vi "Read Tiff File (Bitmiracle libtiff.net)_v2.vi"(8 "error in (no error)":errorcluster, 11 "Input path":path=path "C:/0_DLPGUI_V2/lowResTest.tif") -> (0 "error out":errorcluster, 2 "ImageData":T1)   [LabVIEW 2022 SP3]
doc: "This SubVI is a modified version of the file Read Tiff File.vi that is included in the libtiff2.llb library. The libtiff2.llb was provided by Nico_MPI on the NI LabVIEW discussion forum at http://forums.ni.com/t5/LabVIEW/Labview-libtiff-implementation/td-p/929843/page/2.\n\nRead a multipage TIFF returning an array of images and the total number of frames. This VI closes the file after returning the images array."
uses:
  Classes/TopLevel/Typedefs/TiffImageData--Cluster.ctl
  <vilib>/LVH/i3 JSON/JSON Parsing/Get Object Parameter Files/Get Object Parameter - Object.vi
  <vilib>/LVH/i3 JSON/JSON Parsing/Get Array Value at Index Files/Get Array Value at Index - Array.vi
  C:/Nuget/BitMiracle.LibTiff.NET.2.4.649/lib/net40/BitMiracle.LibTiff.NET.dll
  Nuget/BitMiracle.LibTiff.NET.2.4.649/lib/net40/BitMiracle.LibTiff.NET.dll
  <vilib>/LVH/i3 JSON/i3-json.lvlib
panel:
  out "Numeric":i32
  out "ChannelTargetMaterials":string[](array[string])
  out "MaterialNames":string[](array[string])
  out "error out 2":errorcluster
  out "Subject":string
  out "0 6":T2(plugin-control)
  out "0 5":T2(plugin-control)
  out "0 4":T2(plugin-control)
  out "0 3":T2(plugin-control)
  out "0 2":T2(plugin-control)
  out "ScanLineSize":i32
  out "0":T2(plugin-control)
  out "element 2":i32
  out "element":i32
  # "278x1271"
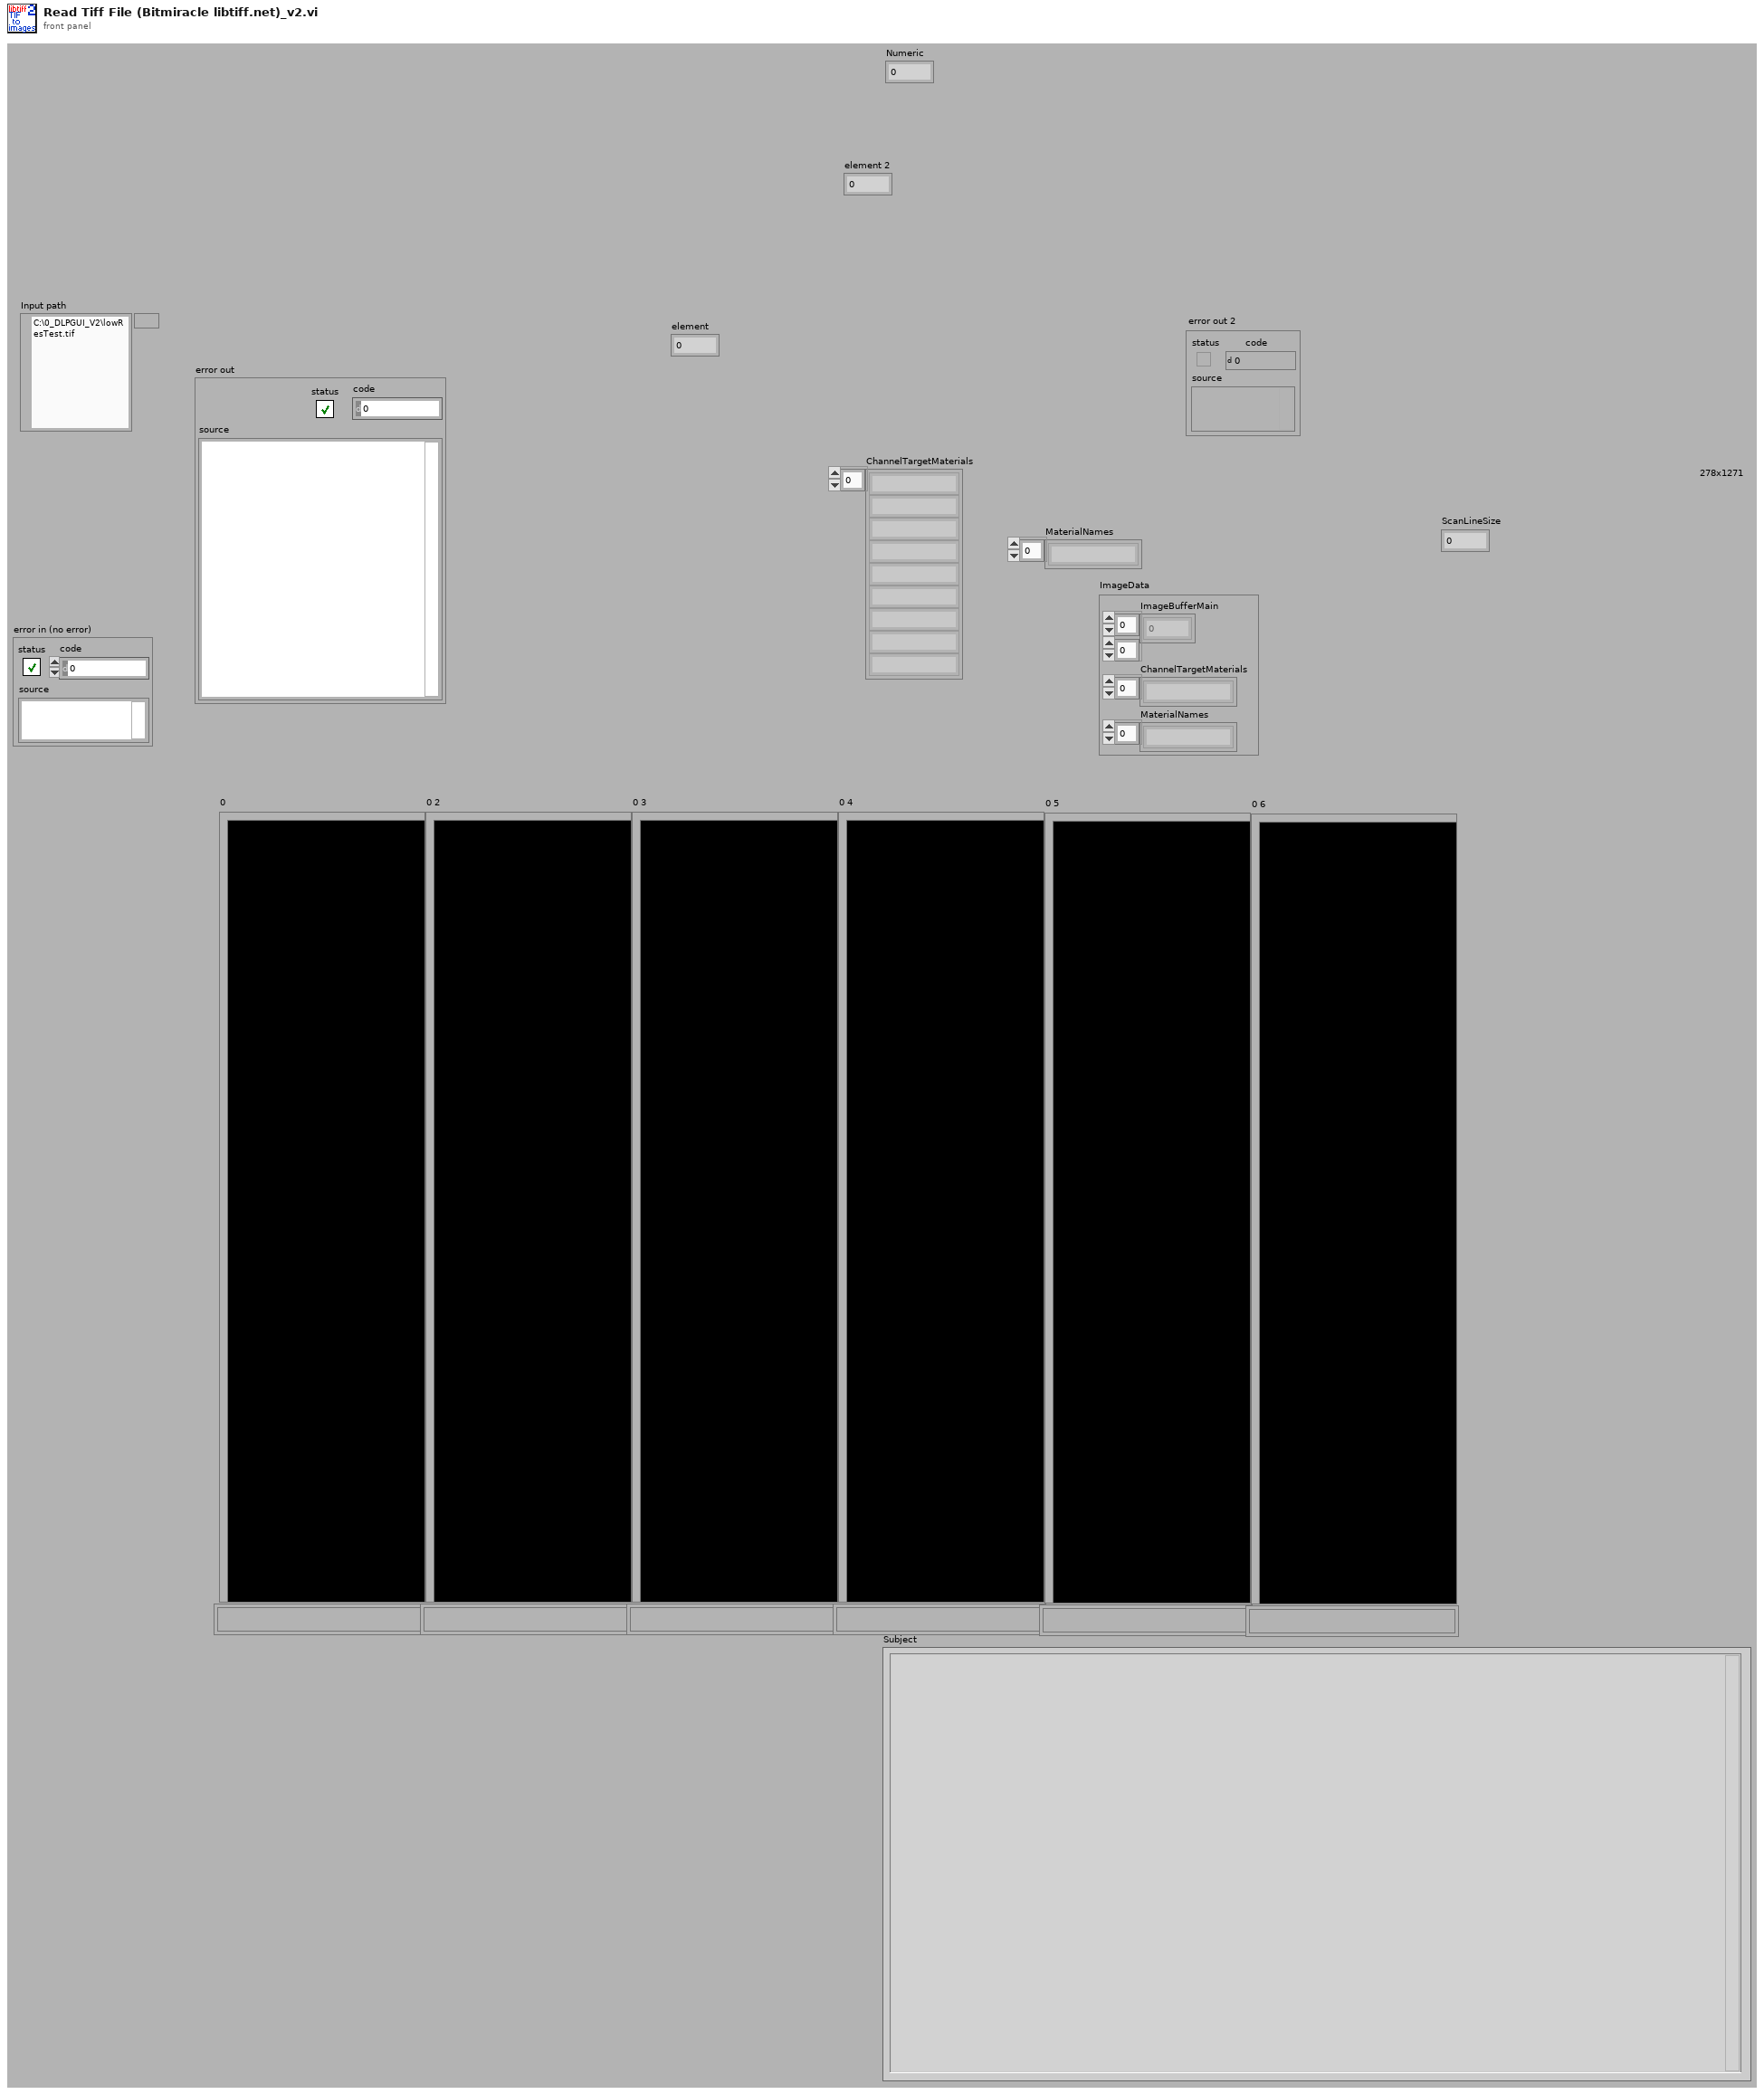
[diagram p1: front panel]
types:
  T1 = typedef "TiffImageData--Cluster.ctl" = cluster{"ImageBufferMain":u8[][], "ChannelTargetMaterials":string[], "MaterialNames":string[]}
  T2 = typedef "IMAQ Image.ctl" = refnum<image>
  T3 = typedef "Image Type" = u32
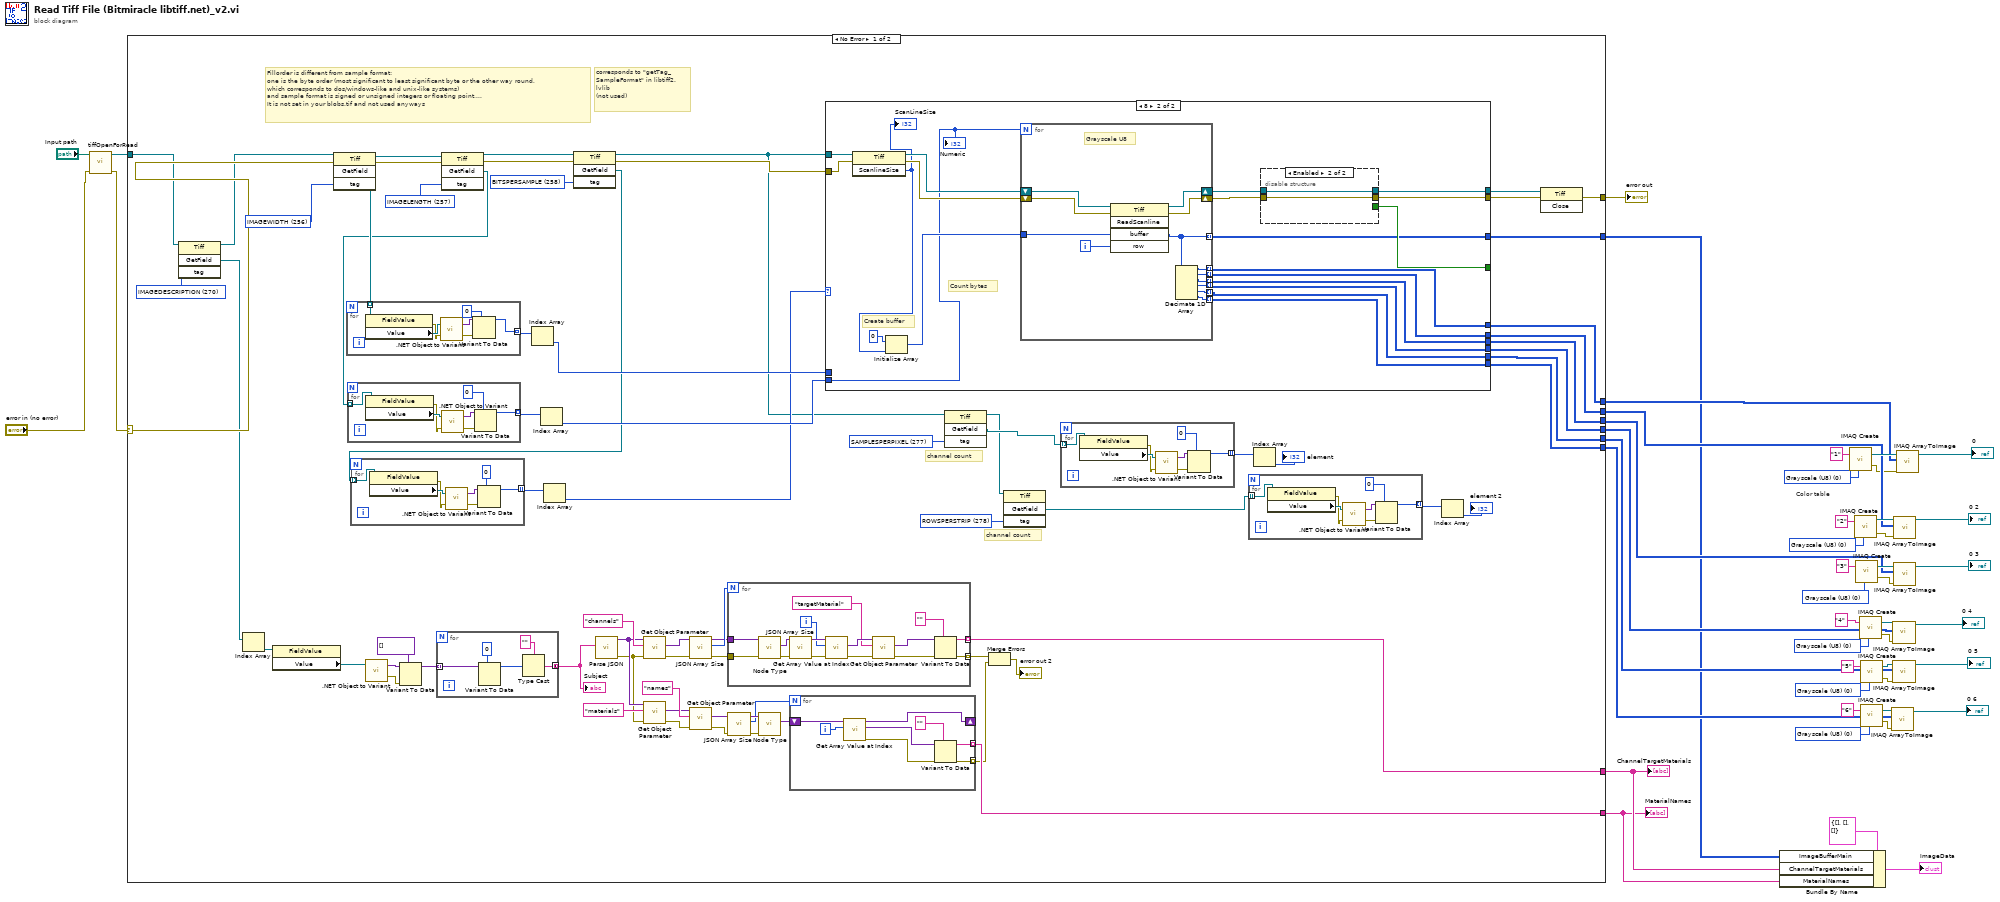
[diagram p0: block diagram]
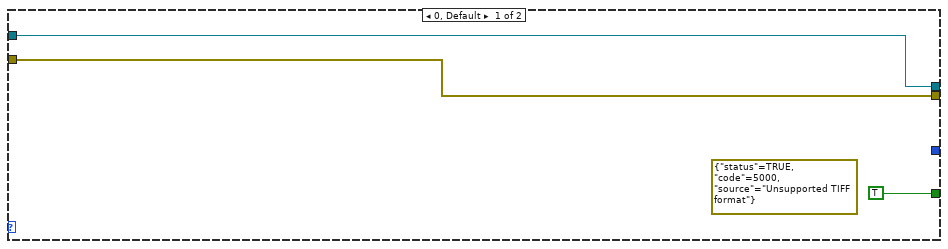
[diagram p2: hidden frame]
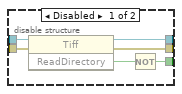
[diagram p3: hidden frame]
diagram:
  w27 = T3 0 items=["Grayscale (U8)", "Grayscale (I16)", "Grayscale (SGL)", "Complex (CSG)", "RGB (U32)", "HSL (U32)", "RGB (U64)", "Grayscale (U16)"] ("Image Type")
  w32 = T3 0 items=["Grayscale (U8)", "Grayscale (I16)", "Grayscale (SGL)", "Complex (CSG)", "RGB (U32)", "HSL (U32)", "RGB (U64)", "Grayscale (U16)"] ("Image Type")
  w29 = T3 0 items=["Grayscale (U8)", "Grayscale (I16)", "Grayscale (SGL)", "Complex (CSG)", "RGB (U32)", "HSL (U32)", "RGB (U64)", "Grayscale (U16)"] ("Image Type")
  w33 = T3 0 items=["Grayscale (U8)", "Grayscale (I16)", "Grayscale (SGL)", "Complex (CSG)", "RGB (U32)", "HSL (U32)", "RGB (U64)", "Grayscale (U16)"] ("Image Type")
  w36 = T3 0 items=["Grayscale (U8)", "Grayscale (I16)", "Grayscale (SGL)", "Complex (CSG)", "RGB (U32)", "HSL (U32)", "RGB (U64)", "Grayscale (U16)"] ("Image Type")
  w40 = T3 0 items=["Grayscale (U8)", "Grayscale (I16)", "Grayscale (SGL)", "Complex (CSG)", "RGB (U32)", "HSL (U32)", "RGB (U64)", "Grayscale (U16)"] ("Image Type")
  # "Color table"
  n1 = call "tiffOpenForRead.vi"("error in (no error)"="error in (no error)", "Path"="Input path") -> ("error out"=w42:errorcluster, "BitMiracle.LibTiff.Classic.Tiff"=w44:refnum<k24>)  [unwired: 8 in]
  n2 = case shown="No Error" w42 {
    selector: w42 -> [w118 w226]
    tunnel: [w114 w226] -> w46
    tunnel: w44 -> [w117 _]
    tunnel: [w113 _] -> w37
    tunnel: [w112 _] -> w24
    tunnel: [w111 _] -> w9
    tunnel: [w110 _] -> w8
    tunnel: [w109 _] -> w7
    tunnel: [w108 _] -> w6
    tunnel: [w107 _] -> w3
    tunnel: [w106 _] -> w2
    tunnel: [w105 _] -> w1
    frame No Error {
      w77 = 270 items=["IGNORE"=0, "SUBFILETYPE"=254, "OSUBFILETYPE"=255, "IMAGEWIDTH"=256, "IMAGELENGTH"=257, "BITSPERSAMPLE"=258, "COMPRESSION"=259, "PHOTOMETRIC"=262, "THRESHHOLDING"=263, "CELLWIDTH"=264, "CELLLENGTH"=265, "FILLORDER"=266, "DOCUMENTNAME"=269, "IMAGEDESCRIPTION"=270, "MAKE"=271, "MODEL"=272, "STRIPOFFSETS"=273, "ORIENTATION"=274, "SAMPLESPERPIXEL"=277, "ROWSPERSTRIP"=278, "STRIPBYTECOUNTS"=279, "MINSAMPLEVALUE"=280, "MAXSAMPLEVALUE"=281, "XRESOLUTION"=282, "YRESOLUTION"=283, "PLANARCONFIG"=284, "PAGENAME"=285, "XPOSITION"=286, "YPOSITION"=287, "FREEOFFSETS"=288, "FREEBYTECOUNTS"=289, "GRAYRESPONSEUNIT"=290, "GRAYRESPONSECURVE"=291, "GROUP3OPTIONS, T4OPTIONS"=292, "GROUP4OPTIONS, T6OPTIONS"=293, "RESOLUTIONUNIT"=296, "PAGENUMBER"=297, "COLORRESPONSEUNIT"=300, "TRANSFERFUNCTION"=301, "SOFTWARE"=305, "DATETIME"=306, "ARTIST"=315, "HOSTCOMPUTER"=316, "PREDICTOR"=317, "WHITEPOINT"=318, "PRIMARYCHROMATICITIES"=319, "COLORMAP"=320, "HALFTONEHINTS"=321, "TILEWIDTH"=322, "TILELENGTH"=323, "TILEOFFSETS"=324, "TILEBYTECOUNTS"=325, "BADFAXLINES"=326, "CLEANFAXDATA"=327, "CONSECUTIVEBADFAXLINES"=328, "SUBIFD"=330, "INKSET"=332, "INKNAMES"=333, "NUMBEROFINKS"=334, "DOTRANGE"=336, "TARGETPRINTER"=337, "EXTRASAMPLES"=338, "SAMPLEFORMAT"=339, "SMINSAMPLEVALUE"=340, "SMAXSAMPLEVALUE"=341, "CLIPPATH"=343, "XCLIPPATHUNITS"=344, "YCLIPPATHUNITS"=345, "INDEXED"=346, "JPEGTABLES"=347, "OPIPROXY"=351, "JPEGPROC"=512, "JPEGIFOFFSET"=513, "JPEGIFBYTECOUNT"=514, "JPEGRESTARTINTERVAL"=515, "JPEGLOSSLESSPREDICTORS"=517, "JPEGPOINTTRANSFORM"=518, "JPEGQTABLES"=519, "JPEGDCTABLES"=520, "JPEGACTABLES"=521, "YCBCRCOEFFICIENTS"=529, "YCBCRSUBSAMPLING"=530, "YCBCRPOSITIONING"=531, "REFERENCEBLACKWHITE"=532, "XMLPACKET"=700, "OPIIMAGEID"=32781, "REFPTS"=32953, "REGIONTACKPOINT"=32954, "REGIONWARPCORNERS"=32955, "REGIONAFFINE"=32956, "MATTEING"=32995, "DATATYPE"=32996, "IMAGEDEPTH"=32997, "TILEDEPTH"=32998, "PIXAR_IMAGEFULLWIDTH"=33300, "PIXAR_IMAGEFULLLENGTH"=33301, "PIXAR_TEXTUREFORMAT"=33302, "PIXAR_WRAPMODES"=33303, "PIXAR_FOVCOT"=33304, "PIXAR_MATRIX_WORLDTOSCREEN"=33305, "PIXAR_MATRIX_WORLDTOCAMERA"=33306, "WRITERSERIALNUMBER"=33405, "COPYRIGHT"=33432, "EXIF_EXPOSURETIME"=33434, "EXIF_FNUMBER"=33437, "GEOTIFF_MODELPIXELSCALETAG"=33550, "RICHTIFFIPTC"=33723, "GEOTIFF_MODELTIEPOINTTAG"=33922, "IT8SITE"=34016, "IT8COLORSEQUENCE"=34017, "IT8HEADER"=34018, "IT8RASTERPADDING"=34019, "IT8BITSPERRUNLENGTH"=34020, "IT8BITSPEREXTENDEDRUNLENGTH"=34021, "IT8COLORTABLE"=34022, "IT8IMAGECOLORINDICATOR"=34023, "IT8BKGCOLORINDICATOR"=34024, "IT8IMAGECOLORVALUE"=34025, "IT8BKGCOLORVALUE"=34026, "IT8PIXELINTENSITYRANGE"=34027, "IT8TRANSPARENCYINDICATOR"=34028, "IT8COLORCHARACTERIZATION"=34029, "IT8HCUSAGE"=34030, "IT8TRAPINDICATOR"=34031, "IT8CMYKEQUIVALENT"=34032, "FRAMECOUNT"=34232, "GEOTIFF_MODELTRANSFORMATIONTAG"=34264, "PHOTOSHOP"=34377, "EXIFIFD"=34665, "ICCPROFILE"=34675, "GEOTIFF_GEOKEYDIRECTORYTAG"=34735, "GEOTIFF_GEODOUBLEPARAMSTAG"=34736, "GEOTIFF_GEOASCIIPARAMSTAG"=34737, "JBIGOPTIONS"=34750, "EXIF_EXPOSUREPROGRAM"=34850, "EXIF_SPECTRALSENSITIVITY"=34852, "GPSIFD"=34853, "EXIF_ISOSPEEDRATINGS"=34855, "EXIF_OECF"=34856, "FAXRECVPARAMS"=34908, "FAXSUBADDRESS"=34909, "FAXRECVTIME"=34910, "FAXDCS"=34911, "FEDEX_EDR"=34929, "EXIF_EXIFVERSION"=36864, "EXIF_DATETIMEORIGINAL"=36867, "EXIF_DATETIMEDIGITIZED"=36868, "EXIF_COMPONENTSCONFIGURATION"=37121, "EXIF_COMPRESSEDBITSPERPIXEL"=37122, "EXIF_SHUTTERSPEEDVALUE"=37377, "EXIF_APERTUREVALUE"=37378, "EXIF_BRIGHTNESSVALUE"=37379, "EXIF_EXPOSUREBIASVALUE"=37380, "EXIF_MAXAPERTUREVALUE"=37381, "EXIF_SUBJECTDISTANCE"=37382, "EXIF_METERINGMODE"=37383, "EXIF_LIGHTSOURCE"=37384, "EXIF_FLASH"=37385, "EXIF_FOCALLENGTH"=37386, "EXIF_SUBJECTAREA"=37396, "STONITS"=37439, "EXIF_MAKERNOTE"=37500, "EXIF_USERCOMMENT"=37510, "EXIF_SUBSECTIME"=37520, "EXIF_SUBSECTIMEORIGINAL"=37521, "EXIF_SUBSECTIMEDIGITIZED"=37522, "EXIF_FLASHPIXVERSION"=40960, "EXIF_COLORSPACE"=40961, "EXIF_PIXELXDIMENSION"=40962, "EXIF_PIXELYDIMENSION"=40963, "EXIF_RELATEDSOUNDFILE"=40964, "INTEROPERABILITYIFD"=40965, "EXIF_FLASHENERGY"=41483, "EXIF_SPATIALFREQUENCYRESPONSE"=41484, "EXIF_FOCALPLANEXRESOLUTION"=41486, "EXIF_FOCALPLANEYRESOLUTION"=41487, "EXIF_FOCALPLANERESOLUTIONUNIT"=41488, "EXIF_SUBJECTLOCATION"=41492, "EXIF_EXPOSUREINDEX"=41493, "EXIF_SENSINGMETHOD"=41495, "EXIF_FILESOURCE"=41728, "EXIF_SCENETYPE"=41729, "EXIF_CFAPATTERN"=41730, "EXIF_CUSTOMRENDERED"=41985, "EXIF_EXPOSUREMODE"=41986, "EXIF_WHITEBALANCE"=41987, "EXIF_DIGITALZOOMRATIO"=41988, "EXIF_FOCALLENGTHIN35MMFILM"=41989, "EXIF_SCENECAPTURETYPE"=41990, "EXIF_GAINCONTROL"=41991, "EXIF_CONTRAST"=41992, "EXIF_SATURATION"=41993, "EXIF_SHARPNESS"=41994, "EXIF_DEVICESETTINGDESCRIPTION"=41995, "EXIF_SUBJECTDISTANCERANGE"=41996, "EXIF_IMAGEUNIQUEID"=42016, "DNGVERSION"=50706, "DNGBACKWARDVERSION"=50707, "UNIQUECAMERAMODEL"=50708, "LOCALIZEDCAMERAMODEL"=50709, "CFAPLANECOLOR"=50710, "CFALAYOUT"=50711, "LINEARIZATIONTABLE"=50712, "BLACKLEVELREPEATDIM"=50713, "BLACKLEVEL"=50714, "BLACKLEVELDELTAH"=50715, "BLACKLEVELDELTAV"=50716, "WHITELEVEL"=50717, "DEFAULTSCALE"=50718, "DEFAULTCROPORIGIN"=50719, "DEFAULTCROPSIZE"=50720, "COLORMATRIX1"=50721, "COLORMATRIX2"=50722, "CAMERACALIBRATION1"=50723, "CAMERACALIBRATION2"=50724, "REDUCTIONMATRIX1"=50725, "REDUCTIONMATRIX2"=50726, "ANALOGBALANCE"=50727, "ASSHOTNEUTRAL"=50728, "ASSHOTWHITEXY"=50729, "BASELINEEXPOSURE"=50730, "BASELINENOISE"=50731, "BASELINESHARPNESS"=50732, "BAYERGREENSPLIT"=50733, "LINEARRESPONSELIMIT"=50734, "CAMERASERIALNUMBER"=50735, "LENSINFO"=50736, "CHROMABLURRADIUS"=50737, "ANTIALIASSTRENGTH"=50738, "SHADOWSCALE"=50739, "DNGPRIVATEDATA"=50740, "MAKERNOTESAFETY"=50741, "CALIBRATIONILLUMINANT1"=50778, "CALIBRATIONILLUMINANT2"=50779, "BESTQUALITYSCALE"=50780, "RAWDATAUNIQUEID"=50781, "ORIGINALRAWFILENAME"=50827, "ORIGINALRAWFILEDATA"=50828, "ACTIVEAREA"=50829, "MASKEDAREAS"=50830, "ASSHOTICCPROFILE"=50831, "ASSHOTPREPROFILEMATRIX"=50832, "CURRENTICCPROFILE"=50833, "CURRENTPREPROFILEMATRIX"=50834, "DCSHUESHIFTVALUES"=65535, "FAXMODE"=65536, "JPEGQUALITY"=65537, "JPEGCOLORMODE"=65538, "JPEGTABLESMODE"=65539, "FAXFILLFUNC"=65540, "PIXARLOGDATAFMT"=65549, "DCSIMAGERTYPE"=65550, "DCSINTERPMODE"=65551, "DCSBALANCEARRAY"=65552, "DCSCORRECTMATRIX"=65553, "DCSGAMMA"=65554, "DCSTOESHOULDERPTS"=65555, "DCSCALIBRATIONFD"=65556, "ZIPQUALITY"=65557, "PIXARLOGQUALITY"=65558, "DCSCLIPRECTANGLE"=65559, "SGILOGDATAFMT"=65560, "SGILOGENCODE"=65561] ("tag")
      w82 = 278 items=["IGNORE"=0, "SUBFILETYPE"=254, "OSUBFILETYPE"=255, "IMAGEWIDTH"=256, "IMAGELENGTH"=257, "BITSPERSAMPLE"=258, "COMPRESSION"=259, "PHOTOMETRIC"=262, "THRESHHOLDING"=263, "CELLWIDTH"=264, "CELLLENGTH"=265, "FILLORDER"=266, "DOCUMENTNAME"=269, "IMAGEDESCRIPTION"=270, "MAKE"=271, "MODEL"=272, "STRIPOFFSETS"=273, "ORIENTATION"=274, "SAMPLESPERPIXEL"=277, "ROWSPERSTRIP"=278, "STRIPBYTECOUNTS"=279, "MINSAMPLEVALUE"=280, "MAXSAMPLEVALUE"=281, "XRESOLUTION"=282, "YRESOLUTION"=283, "PLANARCONFIG"=284, "PAGENAME"=285, "XPOSITION"=286, "YPOSITION"=287, "FREEOFFSETS"=288, "FREEBYTECOUNTS"=289, "GRAYRESPONSEUNIT"=290, "GRAYRESPONSECURVE"=291, "GROUP3OPTIONS, T4OPTIONS"=292, "GROUP4OPTIONS, T6OPTIONS"=293, "RESOLUTIONUNIT"=296, "PAGENUMBER"=297, "COLORRESPONSEUNIT"=300, "TRANSFERFUNCTION"=301, "SOFTWARE"=305, "DATETIME"=306, "ARTIST"=315, "HOSTCOMPUTER"=316, "PREDICTOR"=317, "WHITEPOINT"=318, "PRIMARYCHROMATICITIES"=319, "COLORMAP"=320, "HALFTONEHINTS"=321, "TILEWIDTH"=322, "TILELENGTH"=323, "TILEOFFSETS"=324, "TILEBYTECOUNTS"=325, "BADFAXLINES"=326, "CLEANFAXDATA"=327, "CONSECUTIVEBADFAXLINES"=328, "SUBIFD"=330, "INKSET"=332, "INKNAMES"=333, "NUMBEROFINKS"=334, "DOTRANGE"=336, "TARGETPRINTER"=337, "EXTRASAMPLES"=338, "SAMPLEFORMAT"=339, "SMINSAMPLEVALUE"=340, "SMAXSAMPLEVALUE"=341, "CLIPPATH"=343, "XCLIPPATHUNITS"=344, "YCLIPPATHUNITS"=345, "INDEXED"=346, "JPEGTABLES"=347, "OPIPROXY"=351, "JPEGPROC"=512, "JPEGIFOFFSET"=513, "JPEGIFBYTECOUNT"=514, "JPEGRESTARTINTERVAL"=515, "JPEGLOSSLESSPREDICTORS"=517, "JPEGPOINTTRANSFORM"=518, "JPEGQTABLES"=519, "JPEGDCTABLES"=520, "JPEGACTABLES"=521, "YCBCRCOEFFICIENTS"=529, "YCBCRSUBSAMPLING"=530, "YCBCRPOSITIONING"=531, "REFERENCEBLACKWHITE"=532, "XMLPACKET"=700, "OPIIMAGEID"=32781, "REFPTS"=32953, "REGIONTACKPOINT"=32954, "REGIONWARPCORNERS"=32955, "REGIONAFFINE"=32956, "MATTEING"=32995, "DATATYPE"=32996, "IMAGEDEPTH"=32997, "TILEDEPTH"=32998, "PIXAR_IMAGEFULLWIDTH"=33300, "PIXAR_IMAGEFULLLENGTH"=33301, "PIXAR_TEXTUREFORMAT"=33302, "PIXAR_WRAPMODES"=33303, "PIXAR_FOVCOT"=33304, "PIXAR_MATRIX_WORLDTOSCREEN"=33305, "PIXAR_MATRIX_WORLDTOCAMERA"=33306, "WRITERSERIALNUMBER"=33405, "COPYRIGHT"=33432, "EXIF_EXPOSURETIME"=33434, "EXIF_FNUMBER"=33437, "RICHTIFFIPTC"=33723, "IT8SITE"=34016, "IT8COLORSEQUENCE"=34017, "IT8HEADER"=34018, "IT8RASTERPADDING"=34019, "IT8BITSPERRUNLENGTH"=34020, "IT8BITSPEREXTENDEDRUNLENGTH"=34021, "IT8COLORTABLE"=34022, "IT8IMAGECOLORINDICATOR"=34023, "IT8BKGCOLORINDICATOR"=34024, "IT8IMAGECOLORVALUE"=34025, "IT8BKGCOLORVALUE"=34026, "IT8PIXELINTENSITYRANGE"=34027, "IT8TRANSPARENCYINDICATOR"=34028, "IT8COLORCHARACTERIZATION"=34029, "IT8HCUSAGE"=34030, "IT8TRAPINDICATOR"=34031, "IT8CMYKEQUIVALENT"=34032, "FRAMECOUNT"=34232, "PHOTOSHOP"=34377, "EXIFIFD"=34665, "ICCPROFILE"=34675, "JBIGOPTIONS"=34750, "EXIF_EXPOSUREPROGRAM"=34850, "EXIF_SPECTRALSENSITIVITY"=34852, "GPSIFD"=34853, "EXIF_ISOSPEEDRATINGS"=34855, "EXIF_OECF"=34856, "FAXRECVPARAMS"=34908, "FAXSUBADDRESS"=34909, "FAXRECVTIME"=34910, "FAXDCS"=34911, "FEDEX_EDR"=34929, "EXIF_EXIFVERSION"=36864, "EXIF_DATETIMEORIGINAL"=36867, "EXIF_DATETIMEDIGITIZED"=36868, "EXIF_COMPONENTSCONFIGURATION"=37121, "EXIF_COMPRESSEDBITSPERPIXEL"=37122, "EXIF_SHUTTERSPEEDVALUE"=37377, "EXIF_APERTUREVALUE"=37378, "EXIF_BRIGHTNESSVALUE"=37379, "EXIF_EXPOSUREBIASVALUE"=37380, "EXIF_MAXAPERTUREVALUE"=37381, "EXIF_SUBJECTDISTANCE"=37382, "EXIF_METERINGMODE"=37383, "EXIF_LIGHTSOURCE"=37384, "EXIF_FLASH"=37385, "EXIF_FOCALLENGTH"=37386, "EXIF_SUBJECTAREA"=37396, "STONITS"=37439, "EXIF_MAKERNOTE"=37500, "EXIF_USERCOMMENT"=37510, "EXIF_SUBSECTIME"=37520, "EXIF_SUBSECTIMEORIGINAL"=37521, "EXIF_SUBSECTIMEDIGITIZED"=37522, "EXIF_FLASHPIXVERSION"=40960, "EXIF_COLORSPACE"=40961, "EXIF_PIXELXDIMENSION"=40962, "EXIF_PIXELYDIMENSION"=40963, "EXIF_RELATEDSOUNDFILE"=40964, "INTEROPERABILITYIFD"=40965, "EXIF_FLASHENERGY"=41483, "EXIF_SPATIALFREQUENCYRESPONSE"=41484, "EXIF_FOCALPLANEXRESOLUTION"=41486, "EXIF_FOCALPLANEYRESOLUTION"=41487, "EXIF_FOCALPLANERESOLUTIONUNIT"=41488, "EXIF_SUBJECTLOCATION"=41492, "EXIF_EXPOSUREINDEX"=41493, "EXIF_SENSINGMETHOD"=41495, "EXIF_FILESOURCE"=41728, "EXIF_SCENETYPE"=41729, "EXIF_CFAPATTERN"=41730, "EXIF_CUSTOMRENDERED"=41985, "EXIF_EXPOSUREMODE"=41986, "EXIF_WHITEBALANCE"=41987, "EXIF_DIGITALZOOMRATIO"=41988, "EXIF_FOCALLENGTHIN35MMFILM"=41989, "EXIF_SCENECAPTURETYPE"=41990, "EXIF_GAINCONTROL"=41991, "EXIF_CONTRAST"=41992, "EXIF_SATURATION"=41993, "EXIF_SHARPNESS"=41994, "EXIF_DEVICESETTINGDESCRIPTION"=41995, "EXIF_SUBJECTDISTANCERANGE"=41996, "EXIF_IMAGEUNIQUEID"=42016, "DNGVERSION"=50706, "DNGBACKWARDVERSION"=50707, "UNIQUECAMERAMODEL"=50708, "LOCALIZEDCAMERAMODEL"=50709, "CFAPLANECOLOR"=50710, "CFALAYOUT"=50711, "LINEARIZATIONTABLE"=50712, "BLACKLEVELREPEATDIM"=50713, "BLACKLEVEL"=50714, "BLACKLEVELDELTAH"=50715, "BLACKLEVELDELTAV"=50716, "WHITELEVEL"=50717, "DEFAULTSCALE"=50718, "DEFAULTCROPORIGIN"=50719, "DEFAULTCROPSIZE"=50720, "COLORMATRIX1"=50721, "COLORMATRIX2"=50722, "CAMERACALIBRATION1"=50723, "CAMERACALIBRATION2"=50724, "REDUCTIONMATRIX1"=50725, "REDUCTIONMATRIX2"=50726, "ANALOGBALANCE"=50727, "ASSHOTNEUTRAL"=50728, "ASSHOTWHITEXY"=50729, "BASELINEEXPOSURE"=50730, "BASELINENOISE"=50731, "BASELINESHARPNESS"=50732, "BAYERGREENSPLIT"=50733, "LINEARRESPONSELIMIT"=50734, "CAMERASERIALNUMBER"=50735, "LENSINFO"=50736, "CHROMABLURRADIUS"=50737, "ANTIALIASSTRENGTH"=50738, "SHADOWSCALE"=50739, "DNGPRIVATEDATA"=50740, "MAKERNOTESAFETY"=50741, "CALIBRATIONILLUMINANT1"=50778, "CALIBRATIONILLUMINANT2"=50779, "BESTQUALITYSCALE"=50780, "RAWDATAUNIQUEID"=50781, "ORIGINALRAWFILENAME"=50827, "ORIGINALRAWFILEDATA"=50828, "ACTIVEAREA"=50829, "MASKEDAREAS"=50830, "ASSHOTICCPROFILE"=50831, "ASSHOTPREPROFILEMATRIX"=50832, "CURRENTICCPROFILE"=50833, "CURRENTPREPROFILEMATRIX"=50834, "DCSHUESHIFTVALUES"=65535, "FAXMODE"=65536, "JPEGQUALITY"=65537, "JPEGCOLORMODE"=65538, "JPEGTABLESMODE"=65539, "FAXFILLFUNC"=65540, "PIXARLOGDATAFMT"=65549, "DCSIMAGERTYPE"=65550, "DCSINTERPMODE"=65551, "DCSBALANCEARRAY"=65552, "DCSCORRECTMATRIX"=65553, "DCSGAMMA"=65554, "DCSTOESHOULDERPTS"=65555, "DCSCALIBRATIONFD"=65556, "ZIPQUALITY"=65557, "PIXARLOGQUALITY"=65558, "DCSCLIPRECTANGLE"=65559, "SGILOGDATAFMT"=65560, "SGILOGENCODE"=65561] ("tag")
      w87 = 277 items=["IGNORE"=0, "SUBFILETYPE"=254, "OSUBFILETYPE"=255, "IMAGEWIDTH"=256, "IMAGELENGTH"=257, "BITSPERSAMPLE"=258, "COMPRESSION"=259, "PHOTOMETRIC"=262, "THRESHHOLDING"=263, "CELLWIDTH"=264, "CELLLENGTH"=265, "FILLORDER"=266, "DOCUMENTNAME"=269, "IMAGEDESCRIPTION"=270, "MAKE"=271, "MODEL"=272, "STRIPOFFSETS"=273, "ORIENTATION"=274, "SAMPLESPERPIXEL"=277, "ROWSPERSTRIP"=278, "STRIPBYTECOUNTS"=279, "MINSAMPLEVALUE"=280, "MAXSAMPLEVALUE"=281, "XRESOLUTION"=282, "YRESOLUTION"=283, "PLANARCONFIG"=284, "PAGENAME"=285, "XPOSITION"=286, "YPOSITION"=287, "FREEOFFSETS"=288, "FREEBYTECOUNTS"=289, "GRAYRESPONSEUNIT"=290, "GRAYRESPONSECURVE"=291, "GROUP3OPTIONS, T4OPTIONS"=292, "GROUP4OPTIONS, T6OPTIONS"=293, "RESOLUTIONUNIT"=296, "PAGENUMBER"=297, "COLORRESPONSEUNIT"=300, "TRANSFERFUNCTION"=301, "SOFTWARE"=305, "DATETIME"=306, "ARTIST"=315, "HOSTCOMPUTER"=316, "PREDICTOR"=317, "WHITEPOINT"=318, "PRIMARYCHROMATICITIES"=319, "COLORMAP"=320, "HALFTONEHINTS"=321, "TILEWIDTH"=322, "TILELENGTH"=323, "TILEOFFSETS"=324, "TILEBYTECOUNTS"=325, "BADFAXLINES"=326, "CLEANFAXDATA"=327, "CONSECUTIVEBADFAXLINES"=328, "SUBIFD"=330, "INKSET"=332, "INKNAMES"=333, "NUMBEROFINKS"=334, "DOTRANGE"=336, "TARGETPRINTER"=337, "EXTRASAMPLES"=338, "SAMPLEFORMAT"=339, "SMINSAMPLEVALUE"=340, "SMAXSAMPLEVALUE"=341, "CLIPPATH"=343, "XCLIPPATHUNITS"=344, "YCLIPPATHUNITS"=345, "INDEXED"=346, "JPEGTABLES"=347, "OPIPROXY"=351, "JPEGPROC"=512, "JPEGIFOFFSET"=513, "JPEGIFBYTECOUNT"=514, "JPEGRESTARTINTERVAL"=515, "JPEGLOSSLESSPREDICTORS"=517, "JPEGPOINTTRANSFORM"=518, "JPEGQTABLES"=519, "JPEGDCTABLES"=520, "JPEGACTABLES"=521, "YCBCRCOEFFICIENTS"=529, "YCBCRSUBSAMPLING"=530, "YCBCRPOSITIONING"=531, "REFERENCEBLACKWHITE"=532, "XMLPACKET"=700, "OPIIMAGEID"=32781, "REFPTS"=32953, "REGIONTACKPOINT"=32954, "REGIONWARPCORNERS"=32955, "REGIONAFFINE"=32956, "MATTEING"=32995, "DATATYPE"=32996, "IMAGEDEPTH"=32997, "TILEDEPTH"=32998, "PIXAR_IMAGEFULLWIDTH"=33300, "PIXAR_IMAGEFULLLENGTH"=33301, "PIXAR_TEXTUREFORMAT"=33302, "PIXAR_WRAPMODES"=33303, "PIXAR_FOVCOT"=33304, "PIXAR_MATRIX_WORLDTOSCREEN"=33305, "PIXAR_MATRIX_WORLDTOCAMERA"=33306, "WRITERSERIALNUMBER"=33405, "COPYRIGHT"=33432, "EXIF_EXPOSURETIME"=33434, "EXIF_FNUMBER"=33437, "RICHTIFFIPTC"=33723, "IT8SITE"=34016, "IT8COLORSEQUENCE"=34017, "IT8HEADER"=34018, "IT8RASTERPADDING"=34019, "IT8BITSPERRUNLENGTH"=34020, "IT8BITSPEREXTENDEDRUNLENGTH"=34021, "IT8COLORTABLE"=34022, "IT8IMAGECOLORINDICATOR"=34023, "IT8BKGCOLORINDICATOR"=34024, "IT8IMAGECOLORVALUE"=34025, "IT8BKGCOLORVALUE"=34026, "IT8PIXELINTENSITYRANGE"=34027, "IT8TRANSPARENCYINDICATOR"=34028, "IT8COLORCHARACTERIZATION"=34029, "IT8HCUSAGE"=34030, "IT8TRAPINDICATOR"=34031, "IT8CMYKEQUIVALENT"=34032, "FRAMECOUNT"=34232, "PHOTOSHOP"=34377, "EXIFIFD"=34665, "ICCPROFILE"=34675, "JBIGOPTIONS"=34750, "EXIF_EXPOSUREPROGRAM"=34850, "EXIF_SPECTRALSENSITIVITY"=34852, "GPSIFD"=34853, "EXIF_ISOSPEEDRATINGS"=34855, "EXIF_OECF"=34856, "FAXRECVPARAMS"=34908, "FAXSUBADDRESS"=34909, "FAXRECVTIME"=34910, "FAXDCS"=34911, "FEDEX_EDR"=34929, "EXIF_EXIFVERSION"=36864, "EXIF_DATETIMEORIGINAL"=36867, "EXIF_DATETIMEDIGITIZED"=36868, "EXIF_COMPONENTSCONFIGURATION"=37121, "EXIF_COMPRESSEDBITSPERPIXEL"=37122, "EXIF_SHUTTERSPEEDVALUE"=37377, "EXIF_APERTUREVALUE"=37378, "EXIF_BRIGHTNESSVALUE"=37379, "EXIF_EXPOSUREBIASVALUE"=37380, "EXIF_MAXAPERTUREVALUE"=37381, "EXIF_SUBJECTDISTANCE"=37382, "EXIF_METERINGMODE"=37383, "EXIF_LIGHTSOURCE"=37384, "EXIF_FLASH"=37385, "EXIF_FOCALLENGTH"=37386, "EXIF_SUBJECTAREA"=37396, "STONITS"=37439, "EXIF_MAKERNOTE"=37500, "EXIF_USERCOMMENT"=37510, "EXIF_SUBSECTIME"=37520, "EXIF_SUBSECTIMEORIGINAL"=37521, "EXIF_SUBSECTIMEDIGITIZED"=37522, "EXIF_FLASHPIXVERSION"=40960, "EXIF_COLORSPACE"=40961, "EXIF_PIXELXDIMENSION"=40962, "EXIF_PIXELYDIMENSION"=40963, "EXIF_RELATEDSOUNDFILE"=40964, "INTEROPERABILITYIFD"=40965, "EXIF_FLASHENERGY"=41483, "EXIF_SPATIALFREQUENCYRESPONSE"=41484, "EXIF_FOCALPLANEXRESOLUTION"=41486, "EXIF_FOCALPLANEYRESOLUTION"=41487, "EXIF_FOCALPLANERESOLUTIONUNIT"=41488, "EXIF_SUBJECTLOCATION"=41492, "EXIF_EXPOSUREINDEX"=41493, "EXIF_SENSINGMETHOD"=41495, "EXIF_FILESOURCE"=41728, "EXIF_SCENETYPE"=41729, "EXIF_CFAPATTERN"=41730, "EXIF_CUSTOMRENDERED"=41985, "EXIF_EXPOSUREMODE"=41986, "EXIF_WHITEBALANCE"=41987, "EXIF_DIGITALZOOMRATIO"=41988, "EXIF_FOCALLENGTHIN35MMFILM"=41989, "EXIF_SCENECAPTURETYPE"=41990, "EXIF_GAINCONTROL"=41991, "EXIF_CONTRAST"=41992, "EXIF_SATURATION"=41993, "EXIF_SHARPNESS"=41994, "EXIF_DEVICESETTINGDESCRIPTION"=41995, "EXIF_SUBJECTDISTANCERANGE"=41996, "EXIF_IMAGEUNIQUEID"=42016, "DNGVERSION"=50706, "DNGBACKWARDVERSION"=50707, "UNIQUECAMERAMODEL"=50708, "LOCALIZEDCAMERAMODEL"=50709, "CFAPLANECOLOR"=50710, "CFALAYOUT"=50711, "LINEARIZATIONTABLE"=50712, "BLACKLEVELREPEATDIM"=50713, "BLACKLEVEL"=50714, "BLACKLEVELDELTAH"=50715, "BLACKLEVELDELTAV"=50716, "WHITELEVEL"=50717, "DEFAULTSCALE"=50718, "DEFAULTCROPORIGIN"=50719, "DEFAULTCROPSIZE"=50720, "COLORMATRIX1"=50721, "COLORMATRIX2"=50722, "CAMERACALIBRATION1"=50723, "CAMERACALIBRATION2"=50724, "REDUCTIONMATRIX1"=50725, "REDUCTIONMATRIX2"=50726, "ANALOGBALANCE"=50727, "ASSHOTNEUTRAL"=50728, "ASSHOTWHITEXY"=50729, "BASELINEEXPOSURE"=50730, "BASELINENOISE"=50731, "BASELINESHARPNESS"=50732, "BAYERGREENSPLIT"=50733, "LINEARRESPONSELIMIT"=50734, "CAMERASERIALNUMBER"=50735, "LENSINFO"=50736, "CHROMABLURRADIUS"=50737, "ANTIALIASSTRENGTH"=50738, "SHADOWSCALE"=50739, "DNGPRIVATEDATA"=50740, "MAKERNOTESAFETY"=50741, "CALIBRATIONILLUMINANT1"=50778, "CALIBRATIONILLUMINANT2"=50779, "BESTQUALITYSCALE"=50780, "RAWDATAUNIQUEID"=50781, "ORIGINALRAWFILENAME"=50827, "ORIGINALRAWFILEDATA"=50828, "ACTIVEAREA"=50829, "MASKEDAREAS"=50830, "ASSHOTICCPROFILE"=50831, "ASSHOTPREPROFILEMATRIX"=50832, "CURRENTICCPROFILE"=50833, "CURRENTPREPROFILEMATRIX"=50834, "DCSHUESHIFTVALUES"=65535, "FAXMODE"=65536, "JPEGQUALITY"=65537, "JPEGCOLORMODE"=65538, "JPEGTABLESMODE"=65539, "FAXFILLFUNC"=65540, "PIXARLOGDATAFMT"=65549, "DCSIMAGERTYPE"=65550, "DCSINTERPMODE"=65551, "DCSBALANCEARRAY"=65552, "DCSCORRECTMATRIX"=65553, "DCSGAMMA"=65554, "DCSTOESHOULDERPTS"=65555, "DCSCALIBRATIONFD"=65556, "ZIPQUALITY"=65557, "PIXARLOGQUALITY"=65558, "DCSCLIPRECTANGLE"=65559, "SGILOGDATAFMT"=65560, "SGILOGENCODE"=65561] ("tag")
      w98 = 258 items=["IGNORE"=0, "SUBFILETYPE"=254, "OSUBFILETYPE"=255, "IMAGEWIDTH"=256, "IMAGELENGTH"=257, "BITSPERSAMPLE"=258, "COMPRESSION"=259, "PHOTOMETRIC"=262, "THRESHHOLDING"=263, "CELLWIDTH"=264, "CELLLENGTH"=265, "FILLORDER"=266, "DOCUMENTNAME"=269, "IMAGEDESCRIPTION"=270, "MAKE"=271, "MODEL"=272, "STRIPOFFSETS"=273, "ORIENTATION"=274, "SAMPLESPERPIXEL"=277, "ROWSPERSTRIP"=278, "STRIPBYTECOUNTS"=279, "MINSAMPLEVALUE"=280, "MAXSAMPLEVALUE"=281, "XRESOLUTION"=282, "YRESOLUTION"=283, "PLANARCONFIG"=284, "PAGENAME"=285, "XPOSITION"=286, "YPOSITION"=287, "FREEOFFSETS"=288, "FREEBYTECOUNTS"=289, "GRAYRESPONSEUNIT"=290, "GRAYRESPONSECURVE"=291, "GROUP3OPTIONS, T4OPTIONS"=292, "GROUP4OPTIONS, T6OPTIONS"=293, "RESOLUTIONUNIT"=296, "PAGENUMBER"=297, "COLORRESPONSEUNIT"=300, "TRANSFERFUNCTION"=301, "SOFTWARE"=305, "DATETIME"=306, "ARTIST"=315, "HOSTCOMPUTER"=316, "PREDICTOR"=317, "WHITEPOINT"=318, "PRIMARYCHROMATICITIES"=319, "COLORMAP"=320, "HALFTONEHINTS"=321, "TILEWIDTH"=322, "TILELENGTH"=323, "TILEOFFSETS"=324, "TILEBYTECOUNTS"=325, "BADFAXLINES"=326, "CLEANFAXDATA"=327, "CONSECUTIVEBADFAXLINES"=328, "SUBIFD"=330, "INKSET"=332, "INKNAMES"=333, "NUMBEROFINKS"=334, "DOTRANGE"=336, "TARGETPRINTER"=337, "EXTRASAMPLES"=338, "SAMPLEFORMAT"=339, "SMINSAMPLEVALUE"=340, "SMAXSAMPLEVALUE"=341, "CLIPPATH"=343, "XCLIPPATHUNITS"=344, "YCLIPPATHUNITS"=345, "INDEXED"=346, "JPEGTABLES"=347, "OPIPROXY"=351, "JPEGPROC"=512, "JPEGIFOFFSET"=513, "JPEGIFBYTECOUNT"=514, "JPEGRESTARTINTERVAL"=515, "JPEGLOSSLESSPREDICTORS"=517, "JPEGPOINTTRANSFORM"=518, "JPEGQTABLES"=519, "JPEGDCTABLES"=520, "JPEGACTABLES"=521, "YCBCRCOEFFICIENTS"=529, "YCBCRSUBSAMPLING"=530, "YCBCRPOSITIONING"=531, "REFERENCEBLACKWHITE"=532, "XMLPACKET"=700, "OPIIMAGEID"=32781, "REFPTS"=32953, "REGIONTACKPOINT"=32954, "REGIONWARPCORNERS"=32955, "REGIONAFFINE"=32956, "MATTEING"=32995, "DATATYPE"=32996, "IMAGEDEPTH"=32997, "TILEDEPTH"=32998, "PIXAR_IMAGEFULLWIDTH"=33300, "PIXAR_IMAGEFULLLENGTH"=33301, "PIXAR_TEXTUREFORMAT"=33302, "PIXAR_WRAPMODES"=33303, "PIXAR_FOVCOT"=33304, "PIXAR_MATRIX_WORLDTOSCREEN"=33305, "PIXAR_MATRIX_WORLDTOCAMERA"=33306, "WRITERSERIALNUMBER"=33405, "COPYRIGHT"=33432, "EXIF_EXPOSURETIME"=33434, "EXIF_FNUMBER"=33437, "RICHTIFFIPTC"=33723, "IT8SITE"=34016, "IT8COLORSEQUENCE"=34017, "IT8HEADER"=34018, "IT8RASTERPADDING"=34019, "IT8BITSPERRUNLENGTH"=34020, "IT8BITSPEREXTENDEDRUNLENGTH"=34021, "IT8COLORTABLE"=34022, "IT8IMAGECOLORINDICATOR"=34023, "IT8BKGCOLORINDICATOR"=34024, "IT8IMAGECOLORVALUE"=34025, "IT8BKGCOLORVALUE"=34026, "IT8PIXELINTENSITYRANGE"=34027, "IT8TRANSPARENCYINDICATOR"=34028, "IT8COLORCHARACTERIZATION"=34029, "IT8HCUSAGE"=34030, "IT8TRAPINDICATOR"=34031, "IT8CMYKEQUIVALENT"=34032, "FRAMECOUNT"=34232, "PHOTOSHOP"=34377, "EXIFIFD"=34665, "ICCPROFILE"=34675, "JBIGOPTIONS"=34750, "EXIF_EXPOSUREPROGRAM"=34850, "EXIF_SPECTRALSENSITIVITY"=34852, "GPSIFD"=34853, "EXIF_ISOSPEEDRATINGS"=34855, "EXIF_OECF"=34856, "FAXRECVPARAMS"=34908, "FAXSUBADDRESS"=34909, "FAXRECVTIME"=34910, "FAXDCS"=34911, "FEDEX_EDR"=34929, "EXIF_EXIFVERSION"=36864, "EXIF_DATETIMEORIGINAL"=36867, "EXIF_DATETIMEDIGITIZED"=36868, "EXIF_COMPONENTSCONFIGURATION"=37121, "EXIF_COMPRESSEDBITSPERPIXEL"=37122, "EXIF_SHUTTERSPEEDVALUE"=37377, "EXIF_APERTUREVALUE"=37378, "EXIF_BRIGHTNESSVALUE"=37379, "EXIF_EXPOSUREBIASVALUE"=37380, "EXIF_MAXAPERTUREVALUE"=37381, "EXIF_SUBJECTDISTANCE"=37382, "EXIF_METERINGMODE"=37383, "EXIF_LIGHTSOURCE"=37384, "EXIF_FLASH"=37385, "EXIF_FOCALLENGTH"=37386, "EXIF_SUBJECTAREA"=37396, "STONITS"=37439, "EXIF_MAKERNOTE"=37500, "EXIF_USERCOMMENT"=37510, "EXIF_SUBSECTIME"=37520, "EXIF_SUBSECTIMEORIGINAL"=37521, "EXIF_SUBSECTIMEDIGITIZED"=37522, "EXIF_FLASHPIXVERSION"=40960, "EXIF_COLORSPACE"=40961, "EXIF_PIXELXDIMENSION"=40962, "EXIF_PIXELYDIMENSION"=40963, "EXIF_RELATEDSOUNDFILE"=40964, "INTEROPERABILITYIFD"=40965, "EXIF_FLASHENERGY"=41483, "EXIF_SPATIALFREQUENCYRESPONSE"=41484, "EXIF_FOCALPLANEXRESOLUTION"=41486, "EXIF_FOCALPLANEYRESOLUTION"=41487, "EXIF_FOCALPLANERESOLUTIONUNIT"=41488, "EXIF_SUBJECTLOCATION"=41492, "EXIF_EXPOSUREINDEX"=41493, "EXIF_SENSINGMETHOD"=41495, "EXIF_FILESOURCE"=41728, "EXIF_SCENETYPE"=41729, "EXIF_CFAPATTERN"=41730, "EXIF_CUSTOMRENDERED"=41985, "EXIF_EXPOSUREMODE"=41986, "EXIF_WHITEBALANCE"=41987, "EXIF_DIGITALZOOMRATIO"=41988, "EXIF_FOCALLENGTHIN35MMFILM"=41989, "EXIF_SCENECAPTURETYPE"=41990, "EXIF_GAINCONTROL"=41991, "EXIF_CONTRAST"=41992, "EXIF_SATURATION"=41993, "EXIF_SHARPNESS"=41994, "EXIF_DEVICESETTINGDESCRIPTION"=41995, "EXIF_SUBJECTDISTANCERANGE"=41996, "EXIF_IMAGEUNIQUEID"=42016, "DNGVERSION"=50706, "DNGBACKWARDVERSION"=50707, "UNIQUECAMERAMODEL"=50708, "LOCALIZEDCAMERAMODEL"=50709, "CFAPLANECOLOR"=50710, "CFALAYOUT"=50711, "LINEARIZATIONTABLE"=50712, "BLACKLEVELREPEATDIM"=50713, "BLACKLEVEL"=50714, "BLACKLEVELDELTAH"=50715, "BLACKLEVELDELTAV"=50716, "WHITELEVEL"=50717, "DEFAULTSCALE"=50718, "DEFAULTCROPORIGIN"=50719, "DEFAULTCROPSIZE"=50720, "COLORMATRIX1"=50721, "COLORMATRIX2"=50722, "CAMERACALIBRATION1"=50723, "CAMERACALIBRATION2"=50724, "REDUCTIONMATRIX1"=50725, "REDUCTIONMATRIX2"=50726, "ANALOGBALANCE"=50727, "ASSHOTNEUTRAL"=50728, "ASSHOTWHITEXY"=50729, "BASELINEEXPOSURE"=50730, "BASELINENOISE"=50731, "BASELINESHARPNESS"=50732, "BAYERGREENSPLIT"=50733, "LINEARRESPONSELIMIT"=50734, "CAMERASERIALNUMBER"=50735, "LENSINFO"=50736, "CHROMABLURRADIUS"=50737, "ANTIALIASSTRENGTH"=50738, "SHADOWSCALE"=50739, "DNGPRIVATEDATA"=50740, "MAKERNOTESAFETY"=50741, "CALIBRATIONILLUMINANT1"=50778, "CALIBRATIONILLUMINANT2"=50779, "BESTQUALITYSCALE"=50780, "RAWDATAUNIQUEID"=50781, "ORIGINALRAWFILENAME"=50827, "ORIGINALRAWFILEDATA"=50828, "ACTIVEAREA"=50829, "MASKEDAREAS"=50830, "ASSHOTICCPROFILE"=50831, "ASSHOTPREPROFILEMATRIX"=50832, "CURRENTICCPROFILE"=50833, "CURRENTPREPROFILEMATRIX"=50834, "DCSHUESHIFTVALUES"=65535, "FAXMODE"=65536, "JPEGQUALITY"=65537, "JPEGCOLORMODE"=65538, "JPEGTABLESMODE"=65539, "FAXFILLFUNC"=65540, "PIXARLOGDATAFMT"=65549, "DCSIMAGERTYPE"=65550, "DCSINTERPMODE"=65551, "DCSBALANCEARRAY"=65552, "DCSCORRECTMATRIX"=65553, "DCSGAMMA"=65554, "DCSTOESHOULDERPTS"=65555, "DCSCALIBRATIONFD"=65556, "ZIPQUALITY"=65557, "PIXARLOGQUALITY"=65558, "DCSCLIPRECTANGLE"=65559, "SGILOGDATAFMT"=65560, "SGILOGENCODE"=65561] ("tag")
      w103 = 257 items=["IGNORE"=0, "SUBFILETYPE"=254, "OSUBFILETYPE"=255, "IMAGEWIDTH"=256, "IMAGELENGTH"=257, "BITSPERSAMPLE"=258, "COMPRESSION"=259, "PHOTOMETRIC"=262, "THRESHHOLDING"=263, "CELLWIDTH"=264, "CELLLENGTH"=265, "FILLORDER"=266, "DOCUMENTNAME"=269, "IMAGEDESCRIPTION"=270, "MAKE"=271, "MODEL"=272, "STRIPOFFSETS"=273, "ORIENTATION"=274, "SAMPLESPERPIXEL"=277, "ROWSPERSTRIP"=278, "STRIPBYTECOUNTS"=279, "MINSAMPLEVALUE"=280, "MAXSAMPLEVALUE"=281, "XRESOLUTION"=282, "YRESOLUTION"=283, "PLANARCONFIG"=284, "PAGENAME"=285, "XPOSITION"=286, "YPOSITION"=287, "FREEOFFSETS"=288, "FREEBYTECOUNTS"=289, "GRAYRESPONSEUNIT"=290, "GRAYRESPONSECURVE"=291, "GROUP3OPTIONS, T4OPTIONS"=292, "GROUP4OPTIONS, T6OPTIONS"=293, "RESOLUTIONUNIT"=296, "PAGENUMBER"=297, "COLORRESPONSEUNIT"=300, "TRANSFERFUNCTION"=301, "SOFTWARE"=305, "DATETIME"=306, "ARTIST"=315, "HOSTCOMPUTER"=316, "PREDICTOR"=317, "WHITEPOINT"=318, "PRIMARYCHROMATICITIES"=319, "COLORMAP"=320, "HALFTONEHINTS"=321, "TILEWIDTH"=322, "TILELENGTH"=323, "TILEOFFSETS"=324, "TILEBYTECOUNTS"=325, "BADFAXLINES"=326, "CLEANFAXDATA"=327, "CONSECUTIVEBADFAXLINES"=328, "SUBIFD"=330, "INKSET"=332, "INKNAMES"=333, "NUMBEROFINKS"=334, "DOTRANGE"=336, "TARGETPRINTER"=337, "EXTRASAMPLES"=338, "SAMPLEFORMAT"=339, "SMINSAMPLEVALUE"=340, "SMAXSAMPLEVALUE"=341, "CLIPPATH"=343, "XCLIPPATHUNITS"=344, "YCLIPPATHUNITS"=345, "INDEXED"=346, "JPEGTABLES"=347, "OPIPROXY"=351, "JPEGPROC"=512, "JPEGIFOFFSET"=513, "JPEGIFBYTECOUNT"=514, "JPEGRESTARTINTERVAL"=515, "JPEGLOSSLESSPREDICTORS"=517, "JPEGPOINTTRANSFORM"=518, "JPEGQTABLES"=519, "JPEGDCTABLES"=520, "JPEGACTABLES"=521, "YCBCRCOEFFICIENTS"=529, "YCBCRSUBSAMPLING"=530, "YCBCRPOSITIONING"=531, "REFERENCEBLACKWHITE"=532, "XMLPACKET"=700, "OPIIMAGEID"=32781, "REFPTS"=32953, "REGIONTACKPOINT"=32954, "REGIONWARPCORNERS"=32955, "REGIONAFFINE"=32956, "MATTEING"=32995, "DATATYPE"=32996, "IMAGEDEPTH"=32997, "TILEDEPTH"=32998, "PIXAR_IMAGEFULLWIDTH"=33300, "PIXAR_IMAGEFULLLENGTH"=33301, "PIXAR_TEXTUREFORMAT"=33302, "PIXAR_WRAPMODES"=33303, "PIXAR_FOVCOT"=33304, "PIXAR_MATRIX_WORLDTOSCREEN"=33305, "PIXAR_MATRIX_WORLDTOCAMERA"=33306, "WRITERSERIALNUMBER"=33405, "COPYRIGHT"=33432, "EXIF_EXPOSURETIME"=33434, "EXIF_FNUMBER"=33437, "RICHTIFFIPTC"=33723, "IT8SITE"=34016, "IT8COLORSEQUENCE"=34017, "IT8HEADER"=34018, "IT8RASTERPADDING"=34019, "IT8BITSPERRUNLENGTH"=34020, "IT8BITSPEREXTENDEDRUNLENGTH"=34021, "IT8COLORTABLE"=34022, "IT8IMAGECOLORINDICATOR"=34023, "IT8BKGCOLORINDICATOR"=34024, "IT8IMAGECOLORVALUE"=34025, "IT8BKGCOLORVALUE"=34026, "IT8PIXELINTENSITYRANGE"=34027, "IT8TRANSPARENCYINDICATOR"=34028, "IT8COLORCHARACTERIZATION"=34029, "IT8HCUSAGE"=34030, "IT8TRAPINDICATOR"=34031, "IT8CMYKEQUIVALENT"=34032, "FRAMECOUNT"=34232, "PHOTOSHOP"=34377, "EXIFIFD"=34665, "ICCPROFILE"=34675, "JBIGOPTIONS"=34750, "EXIF_EXPOSUREPROGRAM"=34850, "EXIF_SPECTRALSENSITIVITY"=34852, "GPSIFD"=34853, "EXIF_ISOSPEEDRATINGS"=34855, "EXIF_OECF"=34856, "FAXRECVPARAMS"=34908, "FAXSUBADDRESS"=34909, "FAXRECVTIME"=34910, "FAXDCS"=34911, "FEDEX_EDR"=34929, "EXIF_EXIFVERSION"=36864, "EXIF_DATETIMEORIGINAL"=36867, "EXIF_DATETIMEDIGITIZED"=36868, "EXIF_COMPONENTSCONFIGURATION"=37121, "EXIF_COMPRESSEDBITSPERPIXEL"=37122, "EXIF_SHUTTERSPEEDVALUE"=37377, "EXIF_APERTUREVALUE"=37378, "EXIF_BRIGHTNESSVALUE"=37379, "EXIF_EXPOSUREBIASVALUE"=37380, "EXIF_MAXAPERTUREVALUE"=37381, "EXIF_SUBJECTDISTANCE"=37382, "EXIF_METERINGMODE"=37383, "EXIF_LIGHTSOURCE"=37384, "EXIF_FLASH"=37385, "EXIF_FOCALLENGTH"=37386, "EXIF_SUBJECTAREA"=37396, "STONITS"=37439, "EXIF_MAKERNOTE"=37500, "EXIF_USERCOMMENT"=37510, "EXIF_SUBSECTIME"=37520, "EXIF_SUBSECTIMEORIGINAL"=37521, "EXIF_SUBSECTIMEDIGITIZED"=37522, "EXIF_FLASHPIXVERSION"=40960, "EXIF_COLORSPACE"=40961, "EXIF_PIXELXDIMENSION"=40962, "EXIF_PIXELYDIMENSION"=40963, "EXIF_RELATEDSOUNDFILE"=40964, "INTEROPERABILITYIFD"=40965, "EXIF_FLASHENERGY"=41483, "EXIF_SPATIALFREQUENCYRESPONSE"=41484, "EXIF_FOCALPLANEXRESOLUTION"=41486, "EXIF_FOCALPLANEYRESOLUTION"=41487, "EXIF_FOCALPLANERESOLUTIONUNIT"=41488, "EXIF_SUBJECTLOCATION"=41492, "EXIF_EXPOSUREINDEX"=41493, "EXIF_SENSINGMETHOD"=41495, "EXIF_FILESOURCE"=41728, "EXIF_SCENETYPE"=41729, "EXIF_CFAPATTERN"=41730, "EXIF_CUSTOMRENDERED"=41985, "EXIF_EXPOSUREMODE"=41986, "EXIF_WHITEBALANCE"=41987, "EXIF_DIGITALZOOMRATIO"=41988, "EXIF_FOCALLENGTHIN35MMFILM"=41989, "EXIF_SCENECAPTURETYPE"=41990, "EXIF_GAINCONTROL"=41991, "EXIF_CONTRAST"=41992, "EXIF_SATURATION"=41993, "EXIF_SHARPNESS"=41994, "EXIF_DEVICESETTINGDESCRIPTION"=41995, "EXIF_SUBJECTDISTANCERANGE"=41996, "EXIF_IMAGEUNIQUEID"=42016, "DNGVERSION"=50706, "DNGBACKWARDVERSION"=50707, "UNIQUECAMERAMODEL"=50708, "LOCALIZEDCAMERAMODEL"=50709, "CFAPLANECOLOR"=50710, "CFALAYOUT"=50711, "LINEARIZATIONTABLE"=50712, "BLACKLEVELREPEATDIM"=50713, "BLACKLEVEL"=50714, "BLACKLEVELDELTAH"=50715, "BLACKLEVELDELTAV"=50716, "WHITELEVEL"=50717, "DEFAULTSCALE"=50718, "DEFAULTCROPORIGIN"=50719, "DEFAULTCROPSIZE"=50720, "COLORMATRIX1"=50721, "COLORMATRIX2"=50722, "CAMERACALIBRATION1"=50723, "CAMERACALIBRATION2"=50724, "REDUCTIONMATRIX1"=50725, "REDUCTIONMATRIX2"=50726, "ANALOGBALANCE"=50727, "ASSHOTNEUTRAL"=50728, "ASSHOTWHITEXY"=50729, "BASELINEEXPOSURE"=50730, "BASELINENOISE"=50731, "BASELINESHARPNESS"=50732, "BAYERGREENSPLIT"=50733, "LINEARRESPONSELIMIT"=50734, "CAMERASERIALNUMBER"=50735, "LENSINFO"=50736, "CHROMABLURRADIUS"=50737, "ANTIALIASSTRENGTH"=50738, "SHADOWSCALE"=50739, "DNGPRIVATEDATA"=50740, "MAKERNOTESAFETY"=50741, "CALIBRATIONILLUMINANT1"=50778, "CALIBRATIONILLUMINANT2"=50779, "BESTQUALITYSCALE"=50780, "RAWDATAUNIQUEID"=50781, "ORIGINALRAWFILENAME"=50827, "ORIGINALRAWFILEDATA"=50828, "ACTIVEAREA"=50829, "MASKEDAREAS"=50830, "ASSHOTICCPROFILE"=50831, "ASSHOTPREPROFILEMATRIX"=50832, "CURRENTICCPROFILE"=50833, "CURRENTPREPROFILEMATRIX"=50834, "DCSHUESHIFTVALUES"=65535, "FAXMODE"=65536, "JPEGQUALITY"=65537, "JPEGCOLORMODE"=65538, "JPEGTABLESMODE"=65539, "FAXFILLFUNC"=65540, "PIXARLOGDATAFMT"=65549, "DCSIMAGERTYPE"=65550, "DCSINTERPMODE"=65551, "DCSBALANCEARRAY"=65552, "DCSCORRECTMATRIX"=65553, "DCSGAMMA"=65554, "DCSTOESHOULDERPTS"=65555, "DCSCALIBRATIONFD"=65556, "ZIPQUALITY"=65557, "PIXARLOGQUALITY"=65558, "DCSCLIPRECTANGLE"=65559, "SGILOGDATAFMT"=65560, "SGILOGENCODE"=65561] ("tag")
      w97 = 256 items=["IGNORE"=0, "SUBFILETYPE"=254, "OSUBFILETYPE"=255, "IMAGEWIDTH"=256, "IMAGELENGTH"=257, "BITSPERSAMPLE"=258, "COMPRESSION"=259, "PHOTOMETRIC"=262, "THRESHHOLDING"=263, "CELLWIDTH"=264, "CELLLENGTH"=265, "FILLORDER"=266, "DOCUMENTNAME"=269, "IMAGEDESCRIPTION"=270, "MAKE"=271, "MODEL"=272, "STRIPOFFSETS"=273, "ORIENTATION"=274, "SAMPLESPERPIXEL"=277, "ROWSPERSTRIP"=278, "STRIPBYTECOUNTS"=279, "MINSAMPLEVALUE"=280, "MAXSAMPLEVALUE"=281, "XRESOLUTION"=282, "YRESOLUTION"=283, "PLANARCONFIG"=284, "PAGENAME"=285, "XPOSITION"=286, "YPOSITION"=287, "FREEOFFSETS"=288, "FREEBYTECOUNTS"=289, "GRAYRESPONSEUNIT"=290, "GRAYRESPONSECURVE"=291, "GROUP3OPTIONS, T4OPTIONS"=292, "GROUP4OPTIONS, T6OPTIONS"=293, "RESOLUTIONUNIT"=296, "PAGENUMBER"=297, "COLORRESPONSEUNIT"=300, "TRANSFERFUNCTION"=301, "SOFTWARE"=305, "DATETIME"=306, "ARTIST"=315, "HOSTCOMPUTER"=316, "PREDICTOR"=317, "WHITEPOINT"=318, "PRIMARYCHROMATICITIES"=319, "COLORMAP"=320, "HALFTONEHINTS"=321, "TILEWIDTH"=322, "TILELENGTH"=323, "TILEOFFSETS"=324, "TILEBYTECOUNTS"=325, "BADFAXLINES"=326, "CLEANFAXDATA"=327, "CONSECUTIVEBADFAXLINES"=328, "SUBIFD"=330, "INKSET"=332, "INKNAMES"=333, "NUMBEROFINKS"=334, "DOTRANGE"=336, "TARGETPRINTER"=337, "EXTRASAMPLES"=338, "SAMPLEFORMAT"=339, "SMINSAMPLEVALUE"=340, "SMAXSAMPLEVALUE"=341, "CLIPPATH"=343, "XCLIPPATHUNITS"=344, "YCLIPPATHUNITS"=345, "INDEXED"=346, "JPEGTABLES"=347, "OPIPROXY"=351, "JPEGPROC"=512, "JPEGIFOFFSET"=513, "JPEGIFBYTECOUNT"=514, "JPEGRESTARTINTERVAL"=515, "JPEGLOSSLESSPREDICTORS"=517, "JPEGPOINTTRANSFORM"=518, "JPEGQTABLES"=519, "JPEGDCTABLES"=520, "JPEGACTABLES"=521, "YCBCRCOEFFICIENTS"=529, "YCBCRSUBSAMPLING"=530, "YCBCRPOSITIONING"=531, "REFERENCEBLACKWHITE"=532, "XMLPACKET"=700, "OPIIMAGEID"=32781, "REFPTS"=32953, "REGIONTACKPOINT"=32954, "REGIONWARPCORNERS"=32955, "REGIONAFFINE"=32956, "MATTEING"=32995, "DATATYPE"=32996, "IMAGEDEPTH"=32997, "TILEDEPTH"=32998, "PIXAR_IMAGEFULLWIDTH"=33300, "PIXAR_IMAGEFULLLENGTH"=33301, "PIXAR_TEXTUREFORMAT"=33302, "PIXAR_WRAPMODES"=33303, "PIXAR_FOVCOT"=33304, "PIXAR_MATRIX_WORLDTOSCREEN"=33305, "PIXAR_MATRIX_WORLDTOCAMERA"=33306, "WRITERSERIALNUMBER"=33405, "COPYRIGHT"=33432, "EXIF_EXPOSURETIME"=33434, "EXIF_FNUMBER"=33437, "RICHTIFFIPTC"=33723, "IT8SITE"=34016, "IT8COLORSEQUENCE"=34017, "IT8HEADER"=34018, "IT8RASTERPADDING"=34019, "IT8BITSPERRUNLENGTH"=34020, "IT8BITSPEREXTENDEDRUNLENGTH"=34021, "IT8COLORTABLE"=34022, "IT8IMAGECOLORINDICATOR"=34023, "IT8BKGCOLORINDICATOR"=34024, "IT8IMAGECOLORVALUE"=34025, "IT8BKGCOLORVALUE"=34026, "IT8PIXELINTENSITYRANGE"=34027, "IT8TRANSPARENCYINDICATOR"=34028, "IT8COLORCHARACTERIZATION"=34029, "IT8HCUSAGE"=34030, "IT8TRAPINDICATOR"=34031, "IT8CMYKEQUIVALENT"=34032, "FRAMECOUNT"=34232, "PHOTOSHOP"=34377, "EXIFIFD"=34665, "ICCPROFILE"=34675, "JBIGOPTIONS"=34750, "EXIF_EXPOSUREPROGRAM"=34850, "EXIF_SPECTRALSENSITIVITY"=34852, "GPSIFD"=34853, "EXIF_ISOSPEEDRATINGS"=34855, "EXIF_OECF"=34856, "FAXRECVPARAMS"=34908, "FAXSUBADDRESS"=34909, "FAXRECVTIME"=34910, "FAXDCS"=34911, "FEDEX_EDR"=34929, "EXIF_EXIFVERSION"=36864, "EXIF_DATETIMEORIGINAL"=36867, "EXIF_DATETIMEDIGITIZED"=36868, "EXIF_COMPONENTSCONFIGURATION"=37121, "EXIF_COMPRESSEDBITSPERPIXEL"=37122, "EXIF_SHUTTERSPEEDVALUE"=37377, "EXIF_APERTUREVALUE"=37378, "EXIF_BRIGHTNESSVALUE"=37379, "EXIF_EXPOSUREBIASVALUE"=37380, "EXIF_MAXAPERTUREVALUE"=37381, "EXIF_SUBJECTDISTANCE"=37382, "EXIF_METERINGMODE"=37383, "EXIF_LIGHTSOURCE"=37384, "EXIF_FLASH"=37385, "EXIF_FOCALLENGTH"=37386, "EXIF_SUBJECTAREA"=37396, "STONITS"=37439, "EXIF_MAKERNOTE"=37500, "EXIF_USERCOMMENT"=37510, "EXIF_SUBSECTIME"=37520, "EXIF_SUBSECTIMEORIGINAL"=37521, "EXIF_SUBSECTIMEDIGITIZED"=37522, "EXIF_FLASHPIXVERSION"=40960, "EXIF_COLORSPACE"=40961, "EXIF_PIXELXDIMENSION"=40962, "EXIF_PIXELYDIMENSION"=40963, "EXIF_RELATEDSOUNDFILE"=40964, "INTEROPERABILITYIFD"=40965, "EXIF_FLASHENERGY"=41483, "EXIF_SPATIALFREQUENCYRESPONSE"=41484, "EXIF_FOCALPLANEXRESOLUTION"=41486, "EXIF_FOCALPLANEYRESOLUTION"=41487, "EXIF_FOCALPLANERESOLUTIONUNIT"=41488, "EXIF_SUBJECTLOCATION"=41492, "EXIF_EXPOSUREINDEX"=41493, "EXIF_SENSINGMETHOD"=41495, "EXIF_FILESOURCE"=41728, "EXIF_SCENETYPE"=41729, "EXIF_CFAPATTERN"=41730, "EXIF_CUSTOMRENDERED"=41985, "EXIF_EXPOSUREMODE"=41986, "EXIF_WHITEBALANCE"=41987, "EXIF_DIGITALZOOMRATIO"=41988, "EXIF_FOCALLENGTHIN35MMFILM"=41989, "EXIF_SCENECAPTURETYPE"=41990, "EXIF_GAINCONTROL"=41991, "EXIF_CONTRAST"=41992, "EXIF_SATURATION"=41993, "EXIF_SHARPNESS"=41994, "EXIF_DEVICESETTINGDESCRIPTION"=41995, "EXIF_SUBJECTDISTANCERANGE"=41996, "EXIF_IMAGEUNIQUEID"=42016, "DNGVERSION"=50706, "DNGBACKWARDVERSION"=50707, "UNIQUECAMERAMODEL"=50708, "LOCALIZEDCAMERAMODEL"=50709, "CFAPLANECOLOR"=50710, "CFALAYOUT"=50711, "LINEARIZATIONTABLE"=50712, "BLACKLEVELREPEATDIM"=50713, "BLACKLEVEL"=50714, "BLACKLEVELDELTAH"=50715, "BLACKLEVELDELTAV"=50716, "WHITELEVEL"=50717, "DEFAULTSCALE"=50718, "DEFAULTCROPORIGIN"=50719, "DEFAULTCROPSIZE"=50720, "COLORMATRIX1"=50721, "COLORMATRIX2"=50722, "CAMERACALIBRATION1"=50723, "CAMERACALIBRATION2"=50724, "REDUCTIONMATRIX1"=50725, "REDUCTIONMATRIX2"=50726, "ANALOGBALANCE"=50727, "ASSHOTNEUTRAL"=50728, "ASSHOTWHITEXY"=50729, "BASELINEEXPOSURE"=50730, "BASELINENOISE"=50731, "BASELINESHARPNESS"=50732, "BAYERGREENSPLIT"=50733, "LINEARRESPONSELIMIT"=50734, "CAMERASERIALNUMBER"=50735, "LENSINFO"=50736, "CHROMABLURRADIUS"=50737, "ANTIALIASSTRENGTH"=50738, "SHADOWSCALE"=50739, "DNGPRIVATEDATA"=50740, "MAKERNOTESAFETY"=50741, "CALIBRATIONILLUMINANT1"=50778, "CALIBRATIONILLUMINANT2"=50779, "BESTQUALITYSCALE"=50780, "RAWDATAUNIQUEID"=50781, "ORIGINALRAWFILENAME"=50827, "ORIGINALRAWFILEDATA"=50828, "ACTIVEAREA"=50829, "MASKEDAREAS"=50830, "ASSHOTICCPROFILE"=50831, "ASSHOTPREPROFILEMATRIX"=50832, "CURRENTICCPROFILE"=50833, "CURRENTPREPROFILEMATRIX"=50834, "DCSHUESHIFTVALUES"=65535, "FAXMODE"=65536, "JPEGQUALITY"=65537, "JPEGCOLORMODE"=65538, "JPEGTABLESMODE"=65539, "FAXFILLFUNC"=65540, "PIXARLOGDATAFMT"=65549, "DCSIMAGERTYPE"=65550, "DCSINTERPMODE"=65551, "DCSBALANCEARRAY"=65552, "DCSCORRECTMATRIX"=65553, "DCSGAMMA"=65554, "DCSTOESHOULDERPTS"=65555, "DCSCALIBRATIONFD"=65556, "ZIPQUALITY"=65557, "PIXARLOGQUALITY"=65558, "DCSCLIPRECTANGLE"=65559, "SGILOGDATAFMT"=65560, "SGILOGENCODE"=65561] ("tag")
      # "channel count"
      # "channel count"
      # "Fillorder is different from sample format:\none is the byte order (most significant to least significant byte or the other way round,\nwhich corresponds to dos/windows-like and unix-like systems)\nand sample format is signed or unsigned integers or floating point,...\nIt is not set in your blobs.tif and not used anyways"
      # "corresponds to \"getTag_SampleFormat\" in libtiff2.lvlib\n(not used)"
      n3 = invoke class="Tiff" method="GetField"(reference=w117, "tag"=w77) -> (reference out=w76:refnum<k24>, "GetField"=w75:refnum<k24>[])  [unwired: 2 in, 2 out]
      n4 = Index Array(array=w75) -> (element=w74:refnum<k24>)  [unwired: 1 in]
      n5 = property class="FieldValue"(reference=w74) -> ("Value"=w73:refnum<k24>)  [unwired: 1 in, 2 out]
      n6 = invoke class="Tiff" method="GetField"(reference=w76, error in=w118, "tag"=w97) -> (reference out=w104:refnum<k24>, error out=w99:errorcluster, "GetField"=w96:refnum<k24>[])  [unwired: 1 in, 1 out]
      n7 = for {
        tunnel: w96 -> [w181] mode=indexing
        tunnel: [w175] -> w95 mode=indexing
        n8 = property class="FieldValue"(reference=w181) -> (error out=w179:errorcluster, "Value"=w180:refnum<k24>)  [unwired: 1 in, 1 out]
        n9 = call <vilib>:".NET Object to Variant.vi"("error in (no error)"=w179, ".NET object"=w180) -> ("error out"=w178:errorcluster, "variant"=w177:variant)
        n10 = Variant To Data(error in=w178, type=0, Variant=w177) -> (data=w175:i32)  [unwired: 1 out]
      }
      n11 = call <vilib>:".NET Object to Variant.vi"(".NET object"=w73) -> ("error out"=w47:errorcluster, "variant"=w72:variant)  [unwired: 1 in]
      n12 = Variant To Data(error in=w47, type=variant[] [], Variant=w72) -> (data=w70:variant[])  [unwired: 1 out]
      n13 = for {
        tunnel: w70 -> [w145] mode=indexing
        tunnel: [w142] -> w48 mode=concatenating
        n14 = Variant To Data(type=u8 0, Variant=w145) -> (data=w144:u8)  [unwired: 1 in, 1 out]
        n15 = Type Cast(type="", x=w144) -> (*(type *) &x=w142:string)
      }
      "Subject" <- w48
      n16 = invoke class="Tiff" method="GetField"(reference=w104, error in=w99, "tag"=w103) -> (reference out=w102:refnum<k24>, error out=w100:errorcluster, "GetField"=w92:refnum<k24>[])  [unwired: 1 in, 1 out]
      n17 = for {
        tunnel: [w169] -> w93 mode=indexing
        tunnel: w92 -> [w168] mode=indexing
        n18 = property class="FieldValue"(reference=w168) -> (error out=w173:errorcluster, "Value"=w174:refnum<k24>)  [unwired: 1 in, 1 out]
        n19 = call <vilib>:".NET Object to Variant.vi"("error in (no error)"=w173, ".NET object"=w174) -> ("error out"=w172:errorcluster, "variant"=w171:variant)
        n20 = Variant To Data(error in=w172, type=0, Variant=w171) -> (data=w169:i32)  [unwired: 1 out]
      }
      n21 = Index Array(array=w95) -> (element=w94:i32)  [unwired: 1 in]
      n22 = Index Array(array=w93) -> (element=w91:i32)  [unwired: 1 in]
      n23 = invoke class="Tiff" method="GetField"(reference=w102, error in=w100, "tag"=w98) -> (reference out=w84:refnum<k24>, error out=w101:errorcluster, "GetField"=w89:refnum<k24>[])  [unwired: 1 in, 1 out]
      n24 = for {
        tunnel: [w162] -> w90 mode=indexing
        tunnel: w89 -> [w161] mode=indexing
        n25 = property class="FieldValue"(reference=w161) -> (error out=w166:errorcluster, "Value"=w167:refnum<k24>)  [unwired: 1 in, 1 out]
        n26 = call <vilib>:".NET Object to Variant.vi"("error in (no error)"=w166, ".NET object"=w167) -> ("error out"=w165:errorcluster, "variant"=w164:variant)
        n27 = Variant To Data(error in=w165, type=0, Variant=w164) -> (data=w162:i32)  [unwired: 1 out]
      }
      n28 = Index Array(array=w90) -> (element=w88:i32)  [unwired: 1 in]
      n29 = call <vilib>:"Parse JSON.vi"("JSON String"=w48) -> ("error out"=w54:errorcluster, "JSON Tree"=w55:variant)  [unwired: 7 in, 2 out]
      n30 = call-poly <vilib>:"Get Object Parameter.vi"("error in (no error)"=w54, "Parameter Name"="channels", "JSON Tree In (JSON Object)"=w55) -> ("error out"=w56:errorcluster, "JSON Object"=w61:variant)  [unwired: 5 in, 2 out]
      n31 = call-poly <vilib>:"Get Object Parameter.vi"("error in (no error)"=w54, "Parameter Name"="materials", "JSON Tree In (JSON Object)"=w55) -> ("error out"=w53:errorcluster, "JSON Object"=w62:variant)  [unwired: 5 in, 2 out]
      n32 = call <vilib>:"JSON Array Size.vi"("error in (no error)"=w56, "JSON Tree In (JSON Array)"=w61) -> ("error out"=w57:errorcluster, "Array Size"=w60:i32, "JSON Tree Passthrough (JSON Array)"=w59:variant)  [unwired: 7 in]
      n33 = call-poly <vilib>:"Get Object Parameter.vi"("error in (no error)"=w53, "Parameter Name"="names", "JSON Tree In (JSON Object)"=w62) -> ("error out"=w52:errorcluster, "JSON Object"=w66:variant)  [unwired: 5 in, 2 out]
      n34 = for {
        N: w60 -> [_]
        tunnel: w59 -> [w133]
        tunnel: [w129] -> w106 mode=indexing
        tunnel: [w120] -> w50 mode=indexing
        tunnel: w57 -> [w119]
        i -> [w125]
        n35 = call <vilib>:"Node Type.vi"("error in (no error)"=w119, "JSON Tree In"=w133) -> ("error out"=w124:errorcluster, "Value"=w132:variant)  [unwired: 5 in, 3 out]
        n36 = call <vilib>:"JSON Array Size.vi"("error in (no error)"=w124, "JSON Tree In (JSON Array)"=w132) -> ("error out"=w123:errorcluster, "JSON Tree Passthrough (JSON Array)"=w131:variant)  [unwired: 7 in, 1 out]
        n37 = call-poly <vilib>:"Get Array Value at Index.vi"("error in (no error)"=w123, "Index"=w125, "JSON Tree In (JSON Array)"=w131) -> ("error out"=w122:errorcluster, "JSON Array"=w130:variant)  [unwired: 5 in, 2 out]
        n38 = call-poly <vilib>:"Get Object Parameter.vi"("error in (no error)"=w122, "Parameter Name"="targetMaterial", "JSON Tree In (JSON Object)"=w130) -> ("error out"=w121:errorcluster, "JSON Object"=w127:variant)  [unwired: 5 in, 2 out]
        n39 = Variant To Data(error in=w121, type="", Variant=w127) -> (data=w129:string, error out=w120:errorcluster)
      }
      n40 = call <vilib>:"JSON Array Size.vi"("error in (no error)"=w52, "JSON Tree In (JSON Array)"=w66) -> ("error out"=w58:errorcluster, "Array Size"=w63:i32, "JSON Tree Passthrough (JSON Array)"=w65:variant)  [unwired: 7 in]
      n41 = call <vilib>:"Node Type.vi"("error in (no error)"=w58, "JSON Tree In"=w65) -> ("Value"=w64:variant)  [unwired: 5 in, 4 out]
      n42 = for {
        N: w63 -> [_]
        shift-right: [w140] -> _
        shift-left: w64 -> [w141]
        tunnel: [w136] -> w105 mode=indexing
        tunnel: [w134] -> w51 mode=indexing
        i -> [w139]
        n43 = call-poly <vilib>:"Get Array Value at Index.vi"("Index"=w139, "JSON Tree In (JSON Array)"=w141) -> ("error out"=w135:errorcluster, "JSON Array"=w138:variant, "JSON Tree Out Passthrough"=w140:variant)  [unwired: 6 in, 1 out]
        n44 = Variant To Data(error in=w135, type="", Variant=w138) -> (data=w136:string, error out=w134:errorcluster)
      }
      n45 = case shown="8" w88 {
        tunnel: [TRUE w200] -> _
        tunnel: w94 -> [_ _]
        tunnel: w91 -> [_ w193]
        tunnel: [_ w191] -> w108
        tunnel: w84 -> [w183 w203]
        tunnel: w101 -> [w182 w202]
        tunnel: [w182 w198] -> w115
        tunnel: [w183 w196] -> w116
        tunnel: [_ w190] -> w113
        tunnel: [_ w189] -> w112
        tunnel: [_ w188] -> w111
        tunnel: [_ w187] -> w110
        tunnel: [_ w186] -> w109
        tunnel: [_ w185] -> w107
        frame 0, Default {
          (unwired) errorcluster {"status"=TRUE, "code"=5000, "source"="Unsupported TIFF format"} ("error out")
        }
        frame 8 {
          # "Count bytes"
          # "Create buffer"
          n46 = invoke class="Tiff" method="ScanlineSize"(reference=w203, error in=w202) -> (reference out=w195:refnum<k24>, error out=w204:errorcluster, "ScanlineSize"=w192:i32)  [unwired: 1 in]
          "ScanLineSize" <- w192
          n47 = Initialize Array(u8 0 ("element"), w192) -> (w194:u8[])
          n48 = for {
            N: w193 -> [_]
            tunnel: w194 -> [w221]
            shift-right: [w224] -> w199
            shift-left: w204 -> [w222]
            shift-right: [w225] -> w201
            shift-left: w195 -> [w223]
            tunnel: [w219] -> w185 mode=indexing
            tunnel: [w218] -> w190 mode=indexing
            tunnel: [w217] -> w189 mode=indexing
            tunnel: [w216] -> w188 mode=indexing
            tunnel: [w215] -> w187 mode=indexing
            tunnel: [w214] -> w186 mode=indexing
            tunnel: [w213] -> w191 mode=indexing
            i -> [w220]
            # "Grayscale U8"
            n49 = invoke class="Tiff" method="ReadScanline"(reference=w223, error in=w222, "buffer"=w221, "row"=w220) -> (reference out=w225:refnum<k24>, error out=w224:errorcluster, "buffer"=w219:u8[])  [unwired: 1 in, 2 out]
            n50 = Decimate 1D Array(w219) -> (w218:u8[], w217:u8[], w216:u8[], w215:u8[], w214:u8[], w213:u8[])
          }
          n51 = disable-structure shown="Enabled" {
            disable-tunnel: w201 -> [w210 w212]
            disable-tunnel: [w209 _] -> w200
            disable-tunnel: w199 -> [w208 w211]
            disable-tunnel: [w207 w211] -> w198
            disable-tunnel: [w205 w212] -> w196
            frame Disabled {
              n52 = invoke class="Tiff" method="ReadDirectory"(reference=w210, error in=w208) -> (reference out=w205:refnum<k24>, error out=w207:errorcluster, "ReadDirectory"=w206:bool)  [unwired: 1 in]
              n53 = Not(x=w206) -> (.not. x?=w209:bool)
            }
            frame Enabled {
            }
          }
          "Numeric" <- w193
        }
      }
      n54 = invoke class="Tiff" method="GetField"(reference=w84, "tag"=w87) -> (reference out=w81:refnum<k24>, "GetField"=w85:refnum<k24>[])  [unwired: 2 in, 2 out]
      n55 = Merge Errors(w50, w51) -> (→"error out 2":errorcluster)
      n56 = invoke class="Tiff" method="GetField"(reference=w81, "tag"=w82) -> ("GetField"=w78:refnum<k24>[])  [unwired: 2 in, 3 out]
      n57 = for {
        tunnel: [w155] -> w86 mode=indexing
        tunnel: w85 -> [w154] mode=indexing
        n58 = property class="FieldValue"(reference=w154) -> (error out=w159:errorcluster, "Value"=w160:refnum<k24>)  [unwired: 1 in, 1 out]
        n59 = call <vilib>:".NET Object to Variant.vi"("error in (no error)"=w159, ".NET object"=w160) -> ("error out"=w158:errorcluster, "variant"=w157:variant)
        n60 = Variant To Data(error in=w158, type=0, Variant=w157) -> (data=w155:i32)  [unwired: 1 out]
      }
      n61 = for {
        tunnel: [w148] -> w79 mode=indexing
        tunnel: w78 -> [w147] mode=indexing
        n62 = property class="FieldValue"(reference=w147) -> (error out=w152:errorcluster, "Value"=w153:refnum<k24>)  [unwired: 1 in, 1 out]
        n63 = call <vilib>:".NET Object to Variant.vi"("error in (no error)"=w152, ".NET object"=w153) -> ("error out"=w151:errorcluster, "variant"=w150:variant)
        n64 = Variant To Data(error in=w151, type=0, Variant=w150) -> (data=w148:i32)  [unwired: 1 out]
      }
      n65 = Index Array(array=w86) -> (element=→"element":i32)  [unwired: 1 in]
      n66 = Index Array(array=w79) -> (element=→"element 2":i32)  [unwired: 1 in]
      n67 = invoke class="Tiff" method="Close"(reference=w116, error in=w115) -> (error out=w114:errorcluster)  [unwired: 1 in, 2 out]
    }
    frame Error {
    }
  }
  "error out" <- w46
  "ChannelTargetMaterials" <- w2
  "MaterialNames" <- w1
  n68 = Bundle By Name(cluster=T1 {"ImageBufferMain"=[], "ChannelTargetMaterials"=[], "MaterialNames"=[]} ("ImageData"), "ImageBufferMain"=w3, "ChannelTargetMaterials"=w2, "MaterialNames"=w1) -> (→"ImageData":T1)
  n69 = call "IMAQ Create"("Image Name"="1", "Image Type"=w40) -> ("New Image"=w39:T2, "error out"=w22:errorcluster)  [unwired: 3 in]
  n70 = call "IMAQ Create"("Image Name"="2", "Image Type"=w36) -> ("New Image"=w25:T2, "error out"=w23:errorcluster)  [unwired: 3 in]
  n71 = call "IMAQ Create"("Image Name"="3", "Image Type"=w33) -> ("New Image"=w11:T2, "error out"=w10:errorcluster)  [unwired: 3 in]
  n72 = call "IMAQ Create"("Image Name"="4", "Image Type"=w29) -> ("New Image"=w18:T2, "error out"=w19:errorcluster)  [unwired: 3 in]
  n73 = call "IMAQ Create"("Image Name"="5", "Image Type"=w32) -> ("New Image"=w15:T2, "error out"=w16:errorcluster)  [unwired: 3 in]
  n74 = call "IMAQ Create"("Image Name"="6", "Image Type"=w27) -> ("New Image"=w12:T2, "error out"=w13:errorcluster)  [unwired: 3 in]
  n75 = call "IMAQ ArrayToImage"("error in (no error)"=w13, "Image Pixels (U8)"=w6, "Image"=w12) -> ("Image Out"=→"0 6":T2)  [unwired: 7 in, 1 out]
  n76 = call "IMAQ ArrayToImage"("error in (no error)"=w19, "Image Pixels (U8)"=w8, "Image"=w18) -> ("Image Out"=→"0 4":T2)  [unwired: 7 in, 1 out]
  n77 = call "IMAQ ArrayToImage"("error in (no error)"=w16, "Image Pixels (U8)"=w7, "Image"=w15) -> ("Image Out"=→"0 5":T2)  [unwired: 7 in, 1 out]
  n78 = call "IMAQ ArrayToImage"("error in (no error)"=w23, "Image Pixels (U8)"=w24, "Image"=w25) -> ("Image Out"=→"0 2":T2)  [unwired: 7 in, 1 out]
  n79 = call "IMAQ ArrayToImage"("error in (no error)"=w10, "Image Pixels (U8)"=w9, "Image"=w11) -> ("Image Out"=→"0 3":T2)  [unwired: 7 in, 1 out]
  n80 = call "IMAQ ArrayToImage"("error in (no error)"=w22, "Image Pixels (U8)"=w37, "Image"=w39) -> ("Image Out"=→"0":T2)  [unwired: 7 in, 1 out]
